vi "main_super.vi"() -> ()   [LabVIEW 2019]
uses:
  Skid_Pump_Water/Padrao_cluster_usuario_entrada_bomba_agua.ctl
  \\SERVERPC\Server/padrao_todos_os_dados_SAIDA.ctl
  \\SERVERPC\Server/padrao_UCM.004.EEL.0300_SAIDA.ctl
  \\SERVERPC\Server/padrao_UCM.004.EEL.0200_SAIDA.ctl
  \\SERVERPC\Server/padrao_INTERNO.ctl
  \\SERVERPC\Server/padrao_ADAM_SAIDA.ctl
  Skid_Pump_Kerosene/Cluster_usuario_entrada_K.ctl
  Skid_Medicao/Padrao_cluster_usuario_entrada(med).ctl
  SkidInjection/Cluster_de_usuario_entrada.ctl
  \\SERVERPC\Server/padrao_tipo_dado.ctl
panel:
  out "KPS-FCV-001-R":dbl
  out "WPS-FCV-001-R":dbl
  out "igual?KMS-EVC-001":bool
  out "igual?WMS-EVC-001B":bool
  out "igual?WMS-EVC-001A":bool
  out "T49 M":bool
  in  "KMS-EVC-001":bool
  out "SKM-FC-KF-AUX 2":bool
  out "T26 K":bool
  in  "KPS-FCV-001-W":i16(slide) scale=0.0..100.0
  out "T24 K":bool
  out "T25 K":bool
  out "igual?AMS-ECV-001A":bool
  out "T26":bool
  in  "WPS-FCV-001-W":i16(slide) scale=0.0..100.0
  out "WPS-FCV-001-AUX":bool
  out "T24":bool
  out "T25":bool
  out "SKM-LAM-CTL":bool
  out "T31 M":bool
  out "T32 M":bool
  out "T30 M":bool
  out "Temperatura":dbl[](array[numeric])
  out "Pressão Diferencial":dbl[](array[numeric])
  out "Pressao Absoluta":dbl[](array[numeric])
  out "SKM-FIC-COR-CTL":bool
  out "igual?AMS-EVC-001C":bool
  out "igual?AMS-EVC-001B":bool
  out "Path":string
  out "Confirma SKM-CV-LAM":bool
  out "Confirma SKM-CV-COR":bool
  out "Confirma caminho 1":bool
  in  "AMS-EVC-001C":bool
  in  "AMS-EVC-001B":bool
  in  "AMS-EVC-001A":bool
  out "SKM-TI-LAM":dbl[](array[numeric])
  in  "Controle ar novo 2":i16(slide) scale=0.0..100.0
  in  "Controle ar novo 1":i16(slide) scale=0.0..100.0
  out "Vazao massica":string
  out "P.dif.":string
  out "P.abs.":string
  out "Temp.":string
  out "SKM-PA-TQ":string
  out "SKM-TI-TQ":string
  out "SKM-PA-BAR":string
  out "SKM-FIM-WF":string
  out "SKM-TI-WF":string
  out "SKI-PD-ST":string
  out "SKM-TI-KF":string
  out "SKM-DEN-COR-KF":string
  out "SKM-TI-COR-KF":string
  out "SKM-FIC-COR-KF":string
  in  "FSS-EVC-803":bool
  in  "FSS-EVC-801":bool
  in  "WPS-EVC-008":bool
  in  "WPS-EVC-007":bool
  in  "WPS-EVC-006":bool
  in  "WPS-EVC-005":bool
  out "tempo-super":dbl
  out "aux4":bool
  out "aux3":bool
  out "aux2":bool
  out "aux1":bool
  out "igual?FSS-EVC-611":bool
  out "igual?FSS-EVC-621":bool
  out "igual?SKS-CV-LT1":bool
  out "igual?SKS-CV-BY1":bool
  out "igual?SKS-CV-LT2":bool
  out "igual?SKS-CV-BY2":bool
  in  "CP-Y-601D":bool caption="SKS-CV-004"
  in  "CP-Y-601H":bool
  out "TM6":bool
  out "FSS-EVC-611":bool
  out "FSS-EVC-621":bool
  out "Maximo  W":bool
  out "Minimo  W":bool
  out "FSS-LSL-621":bool
  out "FSS-LSH-621":bool
  out "FSS-LSA-621":bool
  out "FSS-LIT-801":dbl(slide) scale=0.0..100.0
  out "TM10":bool
  out "TM9":bool
  out "TM8":bool
  in  "FSS-EVC-804":bool
  out "TK6":bool
  out "TW6":bool
  out "TK5":bool
  out "TW5":bool
  out "TM5":bool
  out "TM11":bool
  out "TM7":bool
  out "TM4":bool
  out "TM3":bool
  out "TM2":bool
  out "TM1":bool
  in  "FSS-EVC-802":bool
  out "TK2":bool
  out "TW2":bool
  out "TW4":bool
  out "TK1":bool
  out "TK3":bool
  out "TK4":bool
  out "TW3":bool
  out "TW1":bool
  out "FSS-LSH-611":bool
  out "FSS-LSL-611":bool
  out "Minimo K":bool
  out "Maximo K":bool
  out "FSS-LIT-802":dbl(slide) scale=0.0..100.0
  out "FSS-LSA-611":bool
  out "FSS-LSA-801":bool
  out "igual?SKI-CV-ST":bool
  out "igual?SKI-CV-AR":bool
  out "igual?SKI-CV-KF-ST":bool
  out "igual?SKI-CV-WF-ST":bool
  out "igual?SKI-CV-KF-BY1":bool
  out "igual?SKI-CV-BY2":bool
  out "igual?SKI-CV-WF-BY1":bool
  out "SPK-RD-VEL[%]":dbl
  in  "certificado_SPK-PD-P":bool
  in  "TD-SPK-RD-VEL":bool
  out "SPW-RD-VEL[%]":dbl
  out "T15 K":bool
  out "T14 K":bool
  out "T16 K":bool
  out "T23 K":bool
  out "T11 K":bool
  out "T10 K":bool
  out "T9 K":bool
  out "T13 K":bool
  out "T17 K":bool
  out "T18 K":bool
  out "T12 K":bool
  out "T6 K":bool
  out "T1 K":bool
  out "T19 K":bool
  out "T8 K":bool
  out "T22 K":bool
  out "T21 K":bool
  out "T20 K":bool
  out "T5 K":bool
  out "T4 K":bool
  out "T3 K":bool
  out "T7 K":bool
  out "T2 K":bool
  out "SKI-PD-ST":dbl[](array[numeric])
  out "T20 I":bool
  out "T19 I":bool
  out "T18 I":bool
  out "T17 I":bool
  out "T16 I":bool
  out "T15 I":bool
  out "T14 I":bool
  out "T13 I":bool
  out "T11 I":bool
  out "T12 I":bool
  out "T10 I":bool
  out "T9 I":bool
  out "T8 I":bool
  out "T7 I":bool
  out "T6 I":bool
  out "T4 I":bool
  out "T5 I":bool
  out "T3 I":bool
  out "T2 I":bool
  out "T1 I":bool
  in  "FIS-EVC-001":bool
  in  "FIS-EVC-002":bool
  in  "FIS-EVC-031":bool
  in  "FIS-EVC-021":bool
  in  "FIS-EVC-011":bool
  in  "FIS-EVC-022":bool
  in  "FIS-EVC-012":bool
  out "igual?SKM-FC-AR":bool
  out "igual?AMS-EVC-001E":bool
  in  "TD-SKM-TI-COR-AR":bool
  in  "TD-SKM-DEN-COR-KF":bool
  in  "TD-SKM-PD-LAM":bool
  in  "TD-SKM-TI-COR-KF":bool
  in  "TD-SKM-PA-LAM":bool
  in  "TD-SKM-FIC-COR-KF":bool
  in  "TD-SKM-TI-LAM":bool
  in  "TD-SKM-DEN-COR-AR":bool
  in  "TD-SKM-FIC-COR-AR":bool
  in  "WMS-FCV-001":i16(slide) scale=0.0..100.0
  in  "KMS-FCV-001":i16(slide) scale=0.0..100.0
  in  "AMS-FY-004A":i16(slide) scale=0.0..100.0
  in  "AMS-PY-005A":i16(slide) scale=0.0..100.0
  in  "AMS-EVC-003A":bool
  in  "WMS-EVC-001B":bool
  in  "WMS-EVC-001A":bool
  in  "valvula nova 6":bool
  in  "Controle de vazao novo 2-aux":bool
  in  "valvula nova 5":bool
  in  "valvula nova 4":bool
  in  "valvula nova 3":bool
  in  "WMS-FIT-001B":bool
  in  "controle de vazao novo 1-aux":bool
  in  "TANQUE_AR":bool
  out "SKM-PA-BAR":dbl[](array[numeric])
  out "Vazao Massica Ar":dbl[](array[numeric])
  out "WMS-FIT-001A":dbl[](array[numeric])
  out "WMS-TIT-001":dbl[](array[numeric])
  out "KMS-TIT-003":dbl[](array[numeric])
  out "KMS-TIT-002":dbl[](array[numeric])
  out "SKM-DEN-COR-AR":dbl[](array[numeric])
  out "SKM-TI-COR-AR":dbl[](array[numeric])
  out "SKM-FIC-COR-AR":dbl[](array[numeric])
  out "SKM-PD-LAM":dbl[](array[numeric])
  out "SKM-PA-LAM":dbl[](array[numeric])
  out "AMS-PIT-003":dbl[](array[numeric])
  out "SKM-DEN-COR-KF":dbl[](array[numeric])
  out "SKM-TI-COR-KF":dbl[](array[numeric])
  out "SKM-FIC-COR-KF":dbl[](array[numeric])
  out "SKM-TI-KF-CTL":bool
  out "SKM-TI-WF-CTL":bool
  out "SKM-FC-AR-AUX":bool
  out "SKM-FC-WF-AUX":bool
  out "SKM-FIM-WF-CTL":bool
  out "SKM-FC-KF-AUX":bool
  out "SKM-FIC-COR-KF-CTL":bool
  out "SKM-PC-TQ-AUX":bool
  out "T17 M":bool
  out "T48 M":bool
  out "T20 M":bool
  out "T18 M":bool
  out "T19 M":bool
  out "T21 M":bool
  out "T11 M":bool
  out "T10 M":bool
  out "T28 M":bool
  out "T23 M":bool
  out "T27 M":bool
  out "T26 M":bool
  out "T25 M":bool
  out "T47 M":bool
  out "T46 M":bool
  out "T45 M":bool
  out "T41 M":bool
  out "T42 M":bool
  out "T43 M":bool
  out "T44 M":bool
  out "T40 M":bool
  out "T38 M":bool
  out "T37 M":bool
  out "T39 M":bool
  out "T36 M":bool
  out "T35 M":bool
  out "T33 M":bool
  out "T34 M":bool
  out "T29 M":bool
  out "T24 M":bool
  out "T22 M":bool
  out "T12 M":bool
  out "T16 M":bool
  out "T15 M":bool
  out "T14 M":bool
  out "T13 M":bool
  out "T9 M":bool
  out "T8 M":bool
  out "T6 M":bool
  out "T7 M":bool
  out "T5 M":bool
  out "T4 M":bool
  out "T2 M":bool
  out "T3 M":bool
  out "T1 M":bool
  out "igual?SPK-WR-VEL":bool
  out "igual?SPK-WR-ON":bool
  out "igual?SPK-WR-OFF":bool
  out "igual?PID-KF-ON":bool
  out "igual?SPK-CV-008":bool
  out "igual?SPK-CV-007":bool
  out "igual?SPK-CV-006":bool
  out "igual?SPK-CV-005":bool
  out "igual?SPK-CV-004":bool
  out "igual?SPK-CV-003":bool
  out "igual?SPK-CV-002":bool
  out "igual?SPK-CV-001":bool
  in  "SPK-WR-VEL":i32(slide) scale=0.0..100.0
  out "SPK-RD-VEL":dbl(knob) scale=0.0..3500.0
  out "SPK-PD-P":dbl
  out "SPK-RD-TU":dbl
  out "SPK-RD-CRT":dbl
  out "SPK-RD-IA":dbl
  out "SPK-RD-ST":dbl
  out "Inversor Desligado":bool
  out "Inversor Ligado":bool
  out "Bomba K":bool
  in  "PID-KF-ON":bool=TRUE
  in  "KPS-WR-OFF":bool
  in  "KPS-WR-ON":bool
  in  "KPS-EVC-006":bool
  in  "KPS-EVC-005":bool
  in  "KPS-EVC-007":bool
  in  "KPS-EVC-008":bool
  in  "KPS-EVC-003":bool
  in  "KPS-EVC-004":bool
  in  "KPS-EVC-002":bool
  in  "KPS-EVC-001":bool
  out "T15":bool
  out "T14":bool
  out "T16":bool
  out "T23":bool
  out "T11":bool
  out "T10":bool
  out "T9":bool
  out "T13":bool
  out "T17":bool
  out "T18":bool
  out "T12":bool
  out "T6":bool
  out "T1":bool
  out "T19":bool
  out "T8":bool
  out "T22":bool
  out "T21":bool
  out "T20":bool
  out "T5":bool
  out "T4":bool
  out "T3":bool
  out "T7":bool
  out "T2":bool
  out "Inversor desligado":bool
  out "Inversor ligado":bool
  out "Bomba W":bool
  out "igual?SPW-WR-VEL":bool
  out "igual?PID-WF-ON":bool
  out "igual?WPS-EVC-003":bool
  out "igual?WPS-EVC-007":bool
  out "igual?WPS-EVC-006":bool
  out "igual?SPW-WR-OFF":bool
  out "igual?SPW-WR-ON":bool
  out "igual?WPS-EVC-008":bool
  out "igual?WPS-EVC-005":bool
  out "igual?WPS-EVC-004":bool
  out "igual?WPS-EVC-002":bool
  out "igual?WPS-EVC-001":bool
  in  "certificado_SPW-PD-P":bool
  in  "TD-SPW-RD-VEL":bool
  out "SPW-PD-P":dbl
  out "SPW-RD-TU":dbl
  out "SPW-RD-CRT":dbl
  out "SPW-RD-IA":dbl
  out "SPW-RD-ST":dbl
  out "SPW-RD-VEL":dbl(knob) scale=0.0..3500.0
  in  "WPS-EVC-001":bool
  in  "WPS-EVC-004":bool
  in  "PID-WF-ON":bool=TRUE
  in  "WPS-WR-OFF":bool
  in  "WPS-WR-ON":bool
  in  "SPW-WR-VEL":i32(slide) scale=0.0..100.0
  in  "WPS-EVC-003":bool
  in  "WPS-EVC-002":bool
  in  "[ESC/STOP]":bool
  out "Comunicacao Server Client":bool
  out "Status_Comunicacao":string
  in  "Abrir Editor Prioridade":bool
  out "RODANDO TESTE ??":bool
  out "Separador":bool
  # "ALL SKIDS"
  # "MAIN"
  # "[rpm]"
  # "[rpm]"
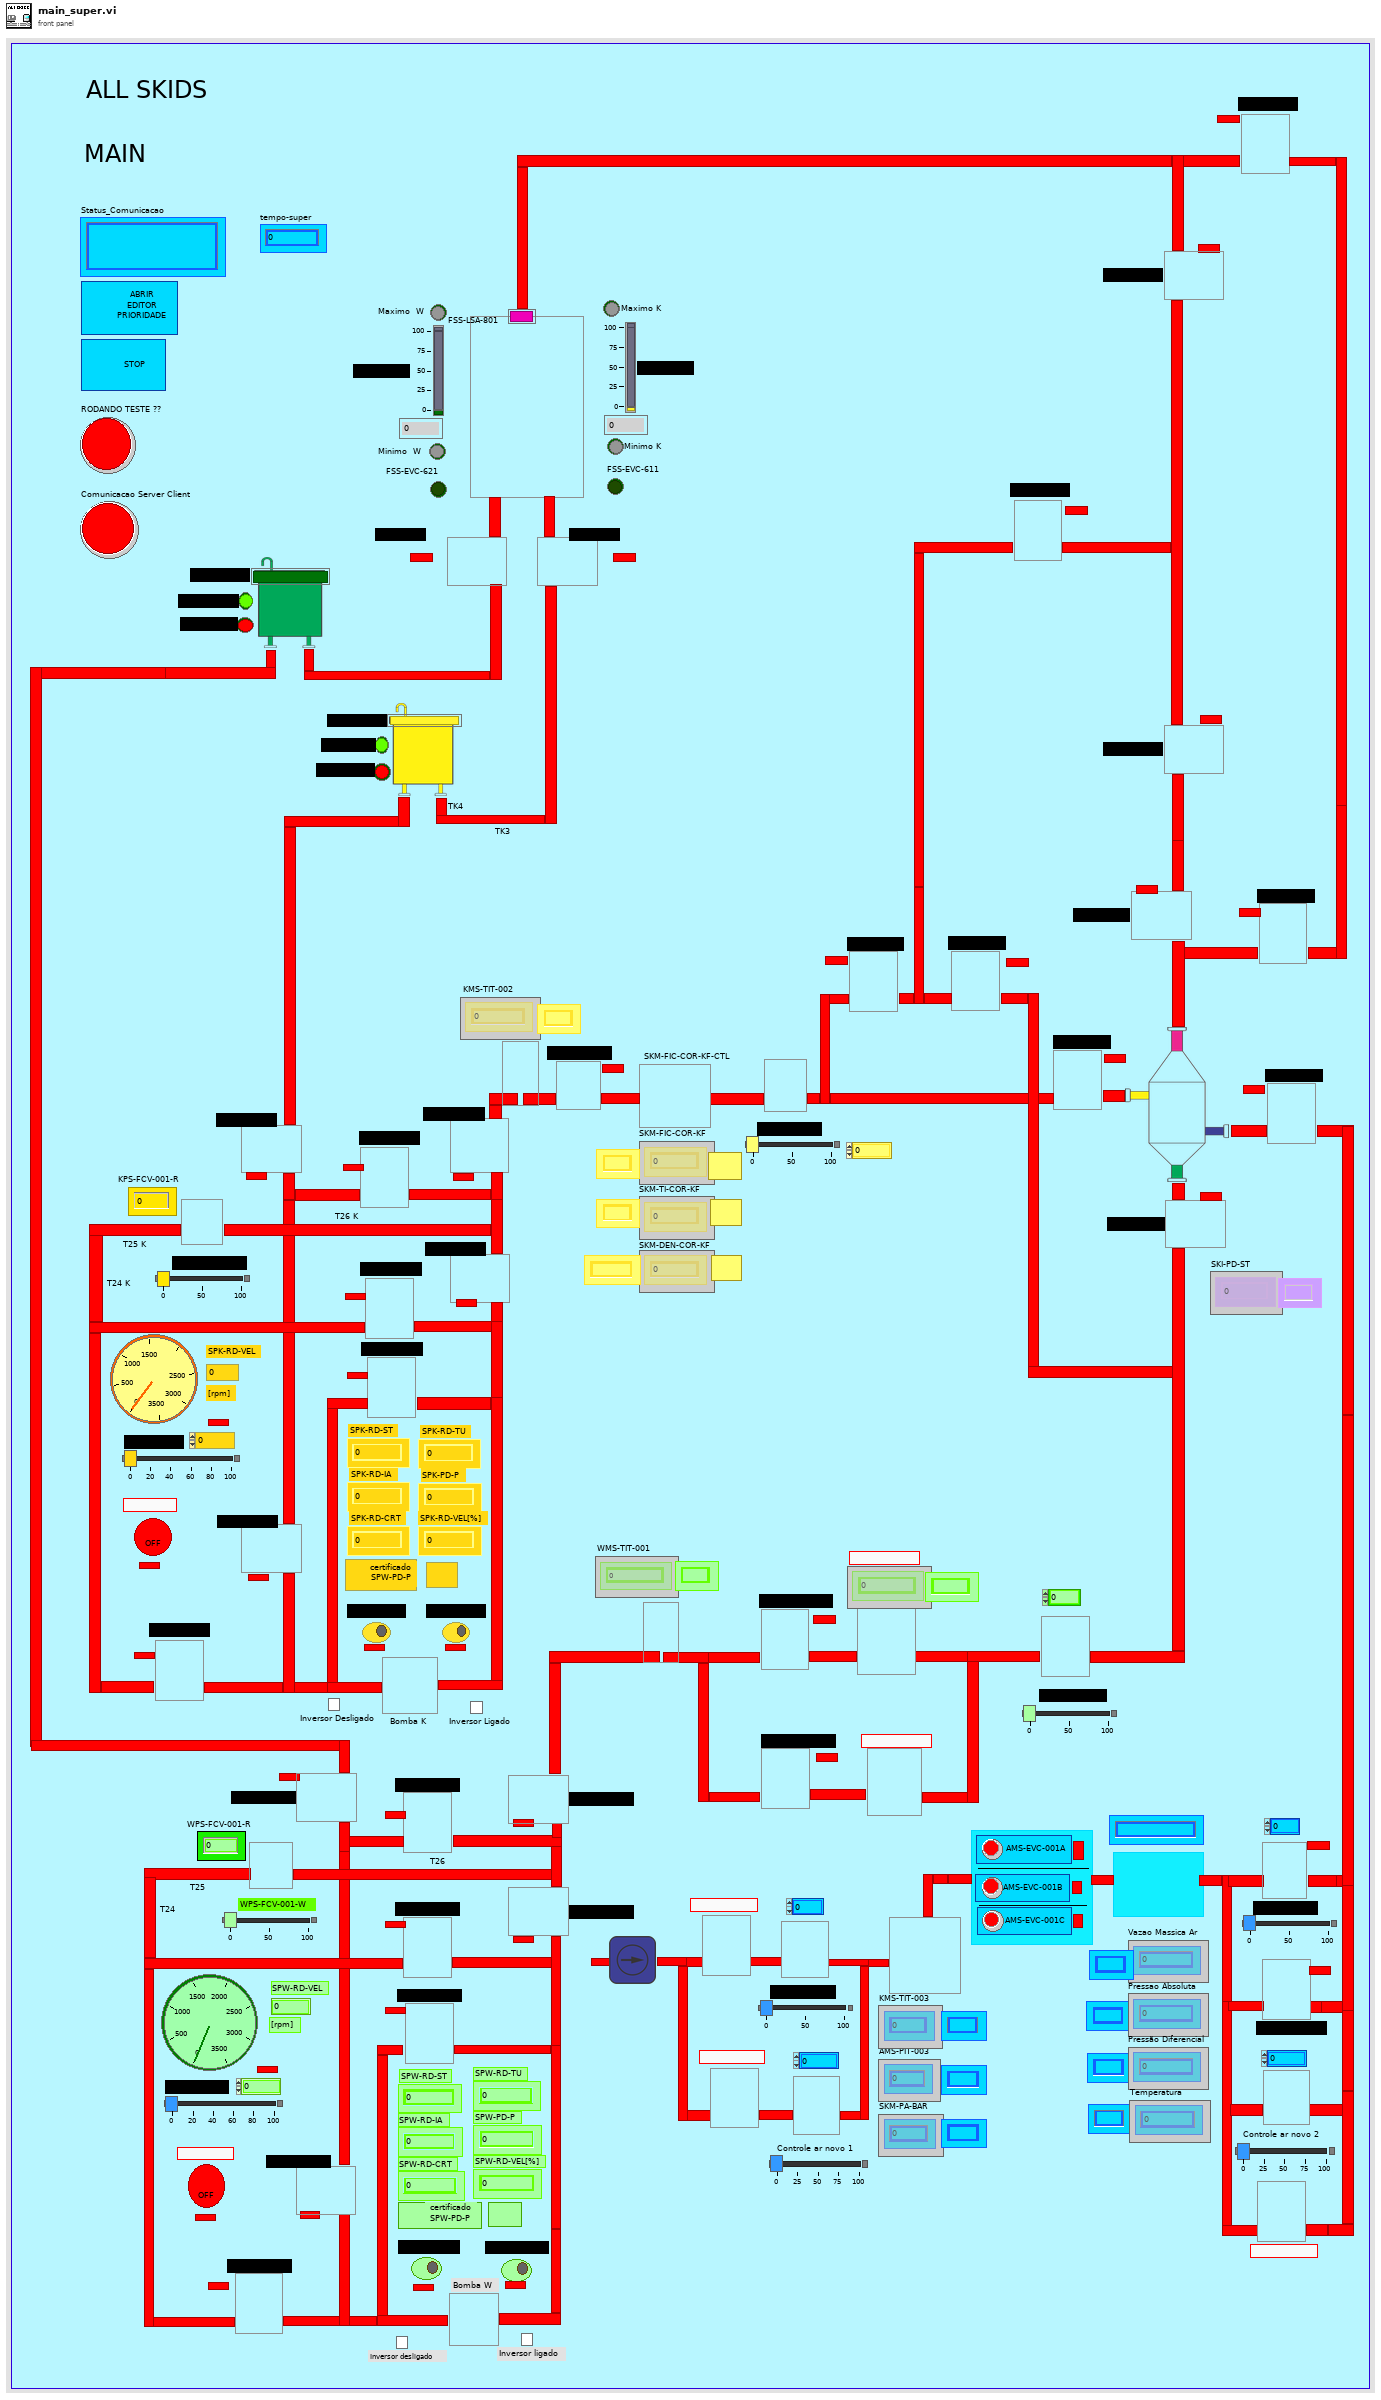
[diagram p1: front panel]
types:
  T1 = typedef "Cluster_de_usuario_entrada.ctl" = cluster{"VI USUARIO":path, "Tipo de Dado_C":T2, "Certificado":bool}
  T2 = typedef "padrao_tipo_dado.ctl" = u16
  T3 = typedef "padrao_todos_os_dados_SAIDA.ctl" = cluster{"UCM.004.EEL.0300_SAIDA":T4, "UCM.004.EEL.0200_SAIDA":T5, "INTERNO":T6, "ADAM_SAIDA":T7}
  T4 = typedef "padrao_UCM.004.EEL.0300_SAIDA.ctl" = cluster{"DIGITAL":cluster{"KPS-EVC-001":bool, "KPS-EVC-002":bool, "KPS-EVC-003":bool, "KPS-EVC-004":bool, "KPS-EVC-005":bool, "KPS-EVC-006":bool, "KPS-EVC-007":bool, "KPS-EVC-008":bool, "WPS-EVC-001":bool, "WPS-EVC-002":bool, "WPS-EVC-003":bool, "WPS-EVC-004":bool, "WPS-EVC-005":bool, "WPS-EVC-006":bool, "WPS-EVC-007":bool, "WPS-EVC-008":bool, "AMS-EVC-001B":bool, "AMS-EVC-003A":bool, "FIS-EVC-031":bool, "FIS-EVC-011":bool, "FIS-EVC-012":bool, "FIS-EVC-021":bool, "FIS-EVC-022":bool, "FIS-EVC-001":bool, "FIS-EVC-002":bool, "KMS-EVC-001":bool, "WMS-EVC-001A":bool, "WMS-EVC-001B":bool, "AMS-EVC-001C":bool, "DG-EVC-001":bool, "DG-EVC-ALL":bool, "PID-PC-TQ-ON":bool, "PID-FC-AR-ON":bool, "PID-WF-ON":bool, "PID-KF-ON":bool, "PID-SA-WF-INV":bool, "PID-SA-KF-INV":bool, "PID-SA-AR-COR":bool, "KPS-WR-ON":bool, "WPS-WR-ON":bool, "KPS-WR-OFF":bool, "WPS-WR-OFF":bool, "AMS-EVC-001A":bool}, "ANALOGICO":cluster{"AMS-PY-005A":i16, "AMS-FY-004A":i16, "WMS-FCV-001":i16, "KMS-FCV-001":i16, "X33 5":i16, "X33 6":i16, "X33 7":i16, "X33 8":i16, "X33 9":i16, "X33 10":i16, "X33 11":i16, "X33 12":i16, "X33 13":i16, "X33 14":i16, "PID-PC-TQ-SP":i16, "PID-FC-AR-SP":i16, "PID-FC-WF-SP":i16, "PID-FC-KF-SP":i16, "PID-INC-WF-SP":i16, "PID-INC-KF-SP":i16, "SPK-WR-VEL":i32, "SPW-WR-VEL":i32, "SKM-FIC-COR-KF-MAX":dbl, "SKM-FIC-COR-KF-MIN":dbl, "SKM-FIC-COR-WF-MAX":dbl, "SKM-FIC-COR-WF-MIN":dbl, "PID-PC-TQ-GP":dbl, "PID-PC-TQ-GI":dbl, "PID-PC-TQ-GD":dbl, "PID-FC-AR-GP":dbl, "PID-FC-AR-GI":dbl, "PID-FC-AR-GD":dbl, "PID-FC-WF-GP":dbl, "PID-FC-WF-GI":dbl, "PID-FC-WF-GD":dbl, "PID-FC-KF-GP":dbl, "PID-FC-KF-GI":dbl, "PID-FC-KF-GD":dbl, "PID-INV-WF-GP":dbl, "PID-INV-WF-GI":dbl, "PID-INV-WF-GD":dbl, "PID-INV-KF-GP":dbl, "PID-INV-KF-GI":dbl, "PID-INV-KF-GD":dbl}}
  T5 = typedef "padrao_UCM.004.EEL.0200_SAIDA.ctl" = cluster{"DIGITAL":cluster{"FSS-EVC-801":bool, "FSS-EVC-802":bool, "FSS-EVC-803":bool, "CP-Y-601D":bool, "CP-Y-601H":bool, "FSS-EVC-804":bool, "SHD-CV-HD":bool, "SHD-CV-ALV":bool, "SHD-ON-OFF":bool, "FSS-EVC-805":bool, "FSS-EVC-806":bool, "X31-12":bool, "X31-13":bool, "X31-14":bool, "X31-15":bool, "X31-16":bool}, "ANALOGICO":cluster{"DG-FCV-801":i16, "X33-2":i16, "FRAM-1100":i16}}
  T6 = typedef "padrao_INTERNO.ctl" = cluster{"DIGITAL":cluster{"ITN-SI-SS-1":bool, "ITN-SI-SS-2":bool, "ITN-SI-SS-3":bool, "ITN-SS-SW-1":bool, "ITN-SS-SK-1":bool, "ITN-SPW-SKM":bool, "ITN-SKMW-SI":bool, "ITN-SKMK-SI":bool, "ITN-SKMA-SI":bool, "ITN-SPK-SKM":bool, "Aplicação apenas de Leitura ??":bool, "SALVAR/AQUISITAR":bool}, "ANALOGICO":cluster{"ITN_Vazao_Massica_Ar":dbl[], "ITN_Vazao_Volumetrica_WF":dbl[], "ITN_Vazao_Massica_KF":dbl[], "ITN_Vazao_Massica_WF":dbl[], "ITN_Vazao_Volumetrica_KF":dbl[], "ITN_Temperatura":dbl[], "ITN_Pressão_Absoluta":dbl[], "ITN_Pressão_Diferencial":dbl[]}, "ALARMES-INTERNOS":cluster{"ALR-AMS-001A+B":bool, "ALR-AMS-001A+C":bool, "ALR-AMS-001B+C":bool, "ALR-AMS-001A+B+C":bool, "ALR-WMS-001A+B":bool}}
  T7 = typedef "padrao_ADAM_SAIDA.ctl" = cluster{"DIGITAL":cluster{"KPS-FCV-001-W":dbl, "WPS-FCV-001-W":dbl, "ADAM-4024-W-2":dbl, "ADAM-4024-W-3":dbl}}
  T8 = typedef "Padrao_cluster_usuario_entrada(med).ctl" = cluster{"VI USUARIO":path, "certificado_SKM-PC-TQ":bool, "certificado_SKM-CV-COR":bool, "certificado_SKM-CV-LAM":bool, "certificado_SKM-CV-JMP":bool, "certificado_SKM-FC-KF":bool, "certificado_SKM-FIC-COR-KF ":bool, "certificado_SKM-FC-WF":bool, "certificado_SKM-FIM-WF":bool, "certificado_SKM-TI-KF":bool, "certificado_SKM-TI-WF":bool, "TD-SKM-TI-COR-AR":bool, "TD-SKM-FIC-COR-AR":bool, "TD-SKM-DEN-COR-AR":bool, "TD-SKM-TI-LAM":bool, "TD-SKM-FIC-COR-KF":bool, "TD-SKM-PA-LAM":bool, "TD-SKM-TI-COR-KF":bool, "TD-SKM-PD-LAM":bool, "TD-SKM-DEN-COR-KF":bool, "certificado_SKM-PA-LAM":bool, "certificado_SKM-PD-LAM":bool, "certificado_SKM-TI-LAM":bool, "certificado_SKM-FIC-COR-AR":bool, "certificado_SKM-PA-BAR":bool}
  T9 = typedef "Cluster_usuario_entrada_K.ctl" = cluster{"File Path Control":path, "certificado_SPK-PD-P":bool, "TD-SPK-RD-VEL":bool, "TD-SPK-RD-IA":bool, "TD-SPK-RD-CRT":bool, "TD-SPK-RD-TU":bool, "TD-SPK-PD-P":bool, "TD-SPK-RD-ST":bool}
  T10 = typedef "Padrao_cluster_usuario_entrada_bomba_agua.ctl" = cluster{"Path Main":path, "certificado_SPW-PD-P":bool, "TD-SPW-RD-VEL":bool, "TD-SPW-RD-IA":bool, "TD-SPW-RD-CRT":bool, "TD-SPW-RD-TU":bool, "TD-SPW-PD-P":bool, "TD-SPW-RD-ST":bool}
  T11 = typedef "padrao_todos_os_dados_ENTRADA.ctl" = cluster{"PAINEL_ADAM_ENTRADA":T12, "todos_os_dados_SAIDA":T3, "UCM.004.EEL.0300_ENTRADA":T13, "UCM.004.EEL.0200_ENTRADA":T14}
  T12 = typedef "padrao_ADAM_ENTRADA.ctl" = cluster{"ANALOGICO":cluster{"KPS-FCV-001-R":dbl, "WPS-FCV-001-R":dbl, "ADAM-4017-01-02":dbl, "ADAM-4017-01-03":dbl, "ADAM-4017-01-04":dbl, "ADAM-4017-01-05":dbl, "ADAM-4017-01-06":dbl, "ADAM-4017-01-07":dbl}, "Laminador_Omega":cluster{"Mode ":string, "Abs. Pressure ":dbl, "Mass Flow":dbl, "Temperature":dbl, "Volumetric Flow":dbl, "Substance ":string}}
  T13 = typedef "padrao_UCM.004.EEL.0300_ENTRADA.ctl" = cluster{"DIGITAL":cluster{"ADAM-ON":bool, "CLP-ON":bool, "KMS-ZT-001":bool, "WMS-ZT-001A":bool, "WMS-ZT-001B":bool, "AMS-ZT-001A":bool, "AMS-ZT-001B":bool, "AMS-ZT-001C":bool, "AMS-ZT-003A":bool, "DG-ZT-001":bool, "DG-ZT-201A":bool, "DG-ZT-201B":bool, "DG-ZT-ON":bool, "DG-ZT-201":bool, "DG-ZT-501":bool, "DG-ZT-701":bool, "KPS-RD-ALR":bool, "KPS-RD-VVT":bool, "KPS-RD-FLL":bool, "WPS-RD-ALR":bool, "WPS-RD-VVT":bool, "WPS-RD-FLL":bool}, "ANALOGICO":cluster{"AMS-PIT-001":dbl[], "AMS-PIT-005":dbl[], "AMS-TIT-005":dbl[], "AMS-PIT-004A":dbl[], "AMS-TIT-004":dbl[], "AMS-PDIT-004A":dbl[], "WMS-TIT-001":dbl[], "WMS-FIT-001B":dbl[], "X32 09":dbl[], "AMS-FIT-004B":dbl[], "WPS-VMS-001":dbl[], "KPS-VMS-001":dbl[], "KMS-TIT-002":dbl[], "WPS-PD-001":dbl[], "KPS-PD-001":dbl[], "X32 16 ":dbl[], "X32 17":dbl[], "X32 18":dbl[], "X32 19":dbl[], "X32 20":dbl[], "X32 21":dbl[], "X32 22":dbl[], "X32 23":dbl[], "X32 24":dbl[], "KPS-RD-ST":dbl[], "WPS-RD-ST":dbl[], "KPS-RD-VEL":dbl[], "WPS-RD-VEL":dbl[], "KPS-RD-IA":dbl[], "WPS-RD-IA":dbl[], "KPS-RD-TU":dbl[], "WPS-RD-TU":dbl[], "KMS-FIT-TI-001":dbl[], "KMS-FIT-DEN-001":dbl[], "KMS-FIT-FIC-001":dbl[], "WMS-FIT-TI-001A":dbl[], "WMS-FIT-DEN-001A":dbl[], "KPS-RD-CRT":dbl[], "WPS-RD-CRT":dbl[], "WMS-FIT-FIC-001A":dbl[]}}
  T14 = typedef "padrao_UCM.004.EEL.0200_ENTRADA.ctl" = cluster{"DIGITAL":cluster{"FSS-LSA-801":bool, "FSS-LSA-621":bool, "FSS-LSA-611":bool, "FSS-LSL-621":bool, "FSS-LSH-621":bool, "FSS-LSL-611":bool, "FSS-LSH-611":bool, "CLP-601-ON":bool, "FSS-ZT-611":bool, "FSS-ZT-621":bool, "X30-11":bool, "X30-12":bool, "DG-ZT-501A":bool, "DG-ZT-501B":bool, "DG-ZT-701A":bool, "DG-ZT-701B":bool}, "ANALOGICO":cluster{"FSS-LIT-802":dbl[], "FSS-LIT-801":dbl[], "SHD-TI-AMB":dbl[], "X32-4":dbl[], "SHD-PD-HD":dbl[], "SHD-PA-JG":dbl[], "X32-7":dbl[], "FRAM-2925":dbl[], "FRAM-2975":dbl[], "FRAM-2976":dbl[], "FRAM-2977":dbl[], "FRAM-2978":dbl[], "FRAM-2979":dbl[], "FRAM-2980":dbl[], "FRAM-2981":dbl[], "FRAM-2982":dbl[], "FRAM-2983":dbl[], "FRAM-2984":dbl[], "FRAM-2985":dbl[], "FRAM-2986":dbl[], "FRAM-2987":dbl[]}}
  T15 = cluster{"igual?SPK-CV-001":bool, "igual?SPK-CV-002":bool, "igual?SPK-CV-003":bool, "igual?SPK-CV-004":bool, "igual?SPK-CV-005":bool, "igual?SPK-CV-006":bool, "igual?SPK-CV-007":bool, "igual?SPK-CV-008":bool, "igual?PID-KF-ON":bool, "igual?SPK-WR-OFF":bool, "igual?SPK-WR-ON":bool, "igual?SPK-WR-VEL":bool, "igual?KPS-FCV-001":bool}
  T16 = typedef "Cluster_usuario_saida_K.ctl" = cluster{"Tubos":cluster{"T1":bool, "T2":bool, "T3":bool, "T4":bool, "T5":bool, "T6":bool, "T7":bool, "T8":bool, "T9":bool, "T10":bool, "T11":bool, "T12":bool, "T13":bool, "T14":bool, "T15":bool, "T16":bool, "T17":bool, "T18":bool, "T19":bool, "T20":bool, "T21":bool, "T22":bool, "T23":bool, "T24":bool, "T25":bool, "T26":bool}, "Leitura_INV":cluster{"SPK-RD-ST":dbl, "SPK-RD-VEL":dbl, "SPK-RD-IA":dbl, "SPK-RD-CRT":dbl, "SPK-RD-TU":dbl, "SPK-PD-P":dbl}, "Inversor":cluster{"Bomba":bool, "Inversor Ligado":bool, "Inversor Desligado":bool}, "Aux":cluster{"SKM-FC-KF-AUX":bool}}
  T17 = cluster{"igual?SPW-CV-001":bool, "igual?SPW-CV-002":bool, "igual?SPW-CV-003":bool, "igual?SPW-CV-004":bool, "igual?SPW-CV-005":bool, "igual?SPW-CV-006":bool, "igual?SPW-CV-007":bool, "igual?SPW-CV-008":bool, "igual?SPW-WR-ON":bool, "igual?SPW-WR-OFF":bool, "igual?PID-WF-ON":bool, "igual?SPW-WR-VEL":bool, "igual?WPS-FVC-001":bool}
  T18 = typedef "Padrao_cluster_usuario_saida_bomba_agua.ctl" = cluster{"Tubos":cluster{"T1":bool, "T2":bool, "T3":bool, "T4":bool, "T5":bool, "T6":bool, "T7":bool, "T8":bool, "T9":bool, "T10":bool, "T11":bool, "T12":bool, "T13":bool, "T14":bool, "T15":bool, "T16":bool, "T17":bool, "T18":bool, "T19":bool, "T20":bool, "T21":bool, "T22":bool, "T23":bool, "T24":bool, "T25":bool, "T26":bool}, "Leitura_INV":cluster{"SPW-RD-ST":dbl, "SPW-RD-VEL":dbl, "SPW-RD-IA":dbl, "SPW-RD-CRT":dbl, "SPW-RD-TU":dbl, "SPW-PD-P":dbl}, "Inversor":cluster{"Bomba":bool, "Inversor Ligado":bool, "Inversor Desligado":bool}, "Aux":cluster{"WPS-FCV-001-AUX":bool}}
  T19 = typedef "Padrao_cluster_usuario_saida_medicao.ctl" = cluster{"Tubos":cluster{"T1":bool, "T2":bool, "T3":bool, "T4":bool, "T5":bool, "T6":bool, "T7":bool, "T8":bool, "T9":bool, "T10":bool, "T11":bool, "T12":bool, "T13":bool, "T14":bool, "T15":bool, "T16":bool, "T17":bool, "T18":bool, "T19":bool, "T20":bool, "T21":bool, "T22":bool, "T23":bool, "T24":bool, "T25":bool, "T26":bool, "T27":bool, "T28":bool, "T29":bool, "T30":bool, "T31":bool, "T32":bool, "T33":bool, "T34":bool, "T35":bool, "T36":bool, "T37":bool, "T38":bool, "T39":bool, "T40":bool, "T41":bool, "T42":bool, "T43":bool, "T44":bool, "T45":bool, "T46":bool, "T47":bool, "T48":bool, "T49":bool}, "Variaveis leitura rapida":cluster{"AMS-PIT-003":dbl[], "SKM-PA-LAM":dbl[], "SKM-TI-LAM":dbl[], "SKM-PD-LAM":dbl[], "WMS-FIT-TI-001A":dbl[], "WMS-FIT-DEN-001A":dbl[], "WMS-FIT-FIC-001A":dbl[], "KMS-FIT-TI-001":dbl[], "KMS-FIT-DEN-001":dbl[], "KMS-FIT-FIC-001":dbl[], "WMS-TIT-001":dbl[], "KMS-TIT-002":dbl[], "KMS-TIT-003":dbl[], "WMS-FIT-001A":dbl[], "Vazao Massica Ar":dbl[], "SKM-PA-BAR":dbl[], "Temperatura":dbl[], "Pressão Absoluta ":dbl[], "Pressão Diferencial":dbl[]}, "Aux":cluster{"SKM-FC-WF-AUX":bool, "SKM-FC-KF-AUX":bool, "SKM-PC-TQ-AUX":bool, "SKM-FC-AR-AUX":bool, "SKM-FIM-WF-CTL":bool, "SKM-FIC-COR-CTL":bool, "SKM-FIC-COR-KF-CTL":bool, "SKM-LAM-CTL":bool, "SKM-TI-KF-CTL":bool, "SKM-TI-TQ-CTL":bool, "SKM-TI-WF-CTL":bool}}
  T20 = cluster{"igual?SKM-FC-WF":bool, "igual?SKM-FC-KF":bool, "igual?SKM-PC-TQ":bool, "igual?SKM-CV-COR":bool, "igual?SKM-CV-LAM":bool, "igual?SKM-CV-JMP":bool, "igual?SKM-FC-AR":bool, "igual?WMS-EVC-001A":bool, "igual?WMS-EVC-001B":bool, "igual?KMS-EVC-001":bool}
  T21 = typedef "Cluster_de_usuario_saida.ctl" = cluster{"Tubos":cluster{"T1":bool, "T 2":bool, "T 3":bool, "T 4":bool, "T 5":bool, "T 6":bool, "T 7":bool, "T 8":bool, "T 9":bool, "T 10":bool, "T 11":bool, "T 12":bool, "T 13":bool, "T 14":bool, "T 15":bool, "T 16":bool, "T 17":bool, "T 18":bool, "T 19":bool, "T 20":bool}, "Leitura":cluster{"SKI-PD-ST":dbl[]}}
  T22 = cluster{"igual?SKI-CV-AR":bool, "igual?SKI-CV-KF-ST":bool, "igual?SKI-CV-KF-BY1":bool, "igual?SKI-CV-WF-ST":bool, "igual?SKI-CV-WF-BY1":bool, "igual?SKI-CV-ST":bool, "igual?SKI-CV-BY2":bool}
  T23 = cluster{"Igual?SKS-CV-BY1":bool, "Igual?SKS-CV-BY2":bool, "Igual?SKS-CV-LT2":bool, "Igual?SKS-CV-TSW":bool, "Igual?SKS-CV-TSK":bool, "Igual?SKS-CV-LT1":bool}
  T24 = cluster{"FSS-LSA-801":bool, "FSS-LSA-621":bool, "FSS-LSA-611":bool, "FSS-LSL-621":bool, "FSS-LSH-621":bool, "FSS-LSL-611":bool, "FSS-LSH-611":bool, "TW2 ":bool, "TK2":bool, "TM5":bool, "TM6":bool, "TM7":bool, "TM8":bool, "TM9":bool, "TM11":bool, "FSS-LIT-801":dbl, "FSS-LIT-802":dbl, "TM10":bool, "Valor minimo atingido K":bool, "Valor maximo atingido K":bool, "Valor maximo atingido W":bool, "Valor minimo atingido W":bool, "TK1":bool, "TW3":bool, "TW4":bool, "TW5":bool, "TW6 ":bool, "TK3":bool, "TK4":bool, "TK5":bool, "TK6":bool, "TM4":bool, "TW1":bool, "FSS-EVC-621":bool, "FSS-EVC-611":bool, "SKS-CV-LT2":bool, "SKS-CV-LT1":bool, "SKS-CV-BY1":bool, "SKS-CV-BY2":bool, "TM1":bool, "TM2":bool, "TM3":bool}
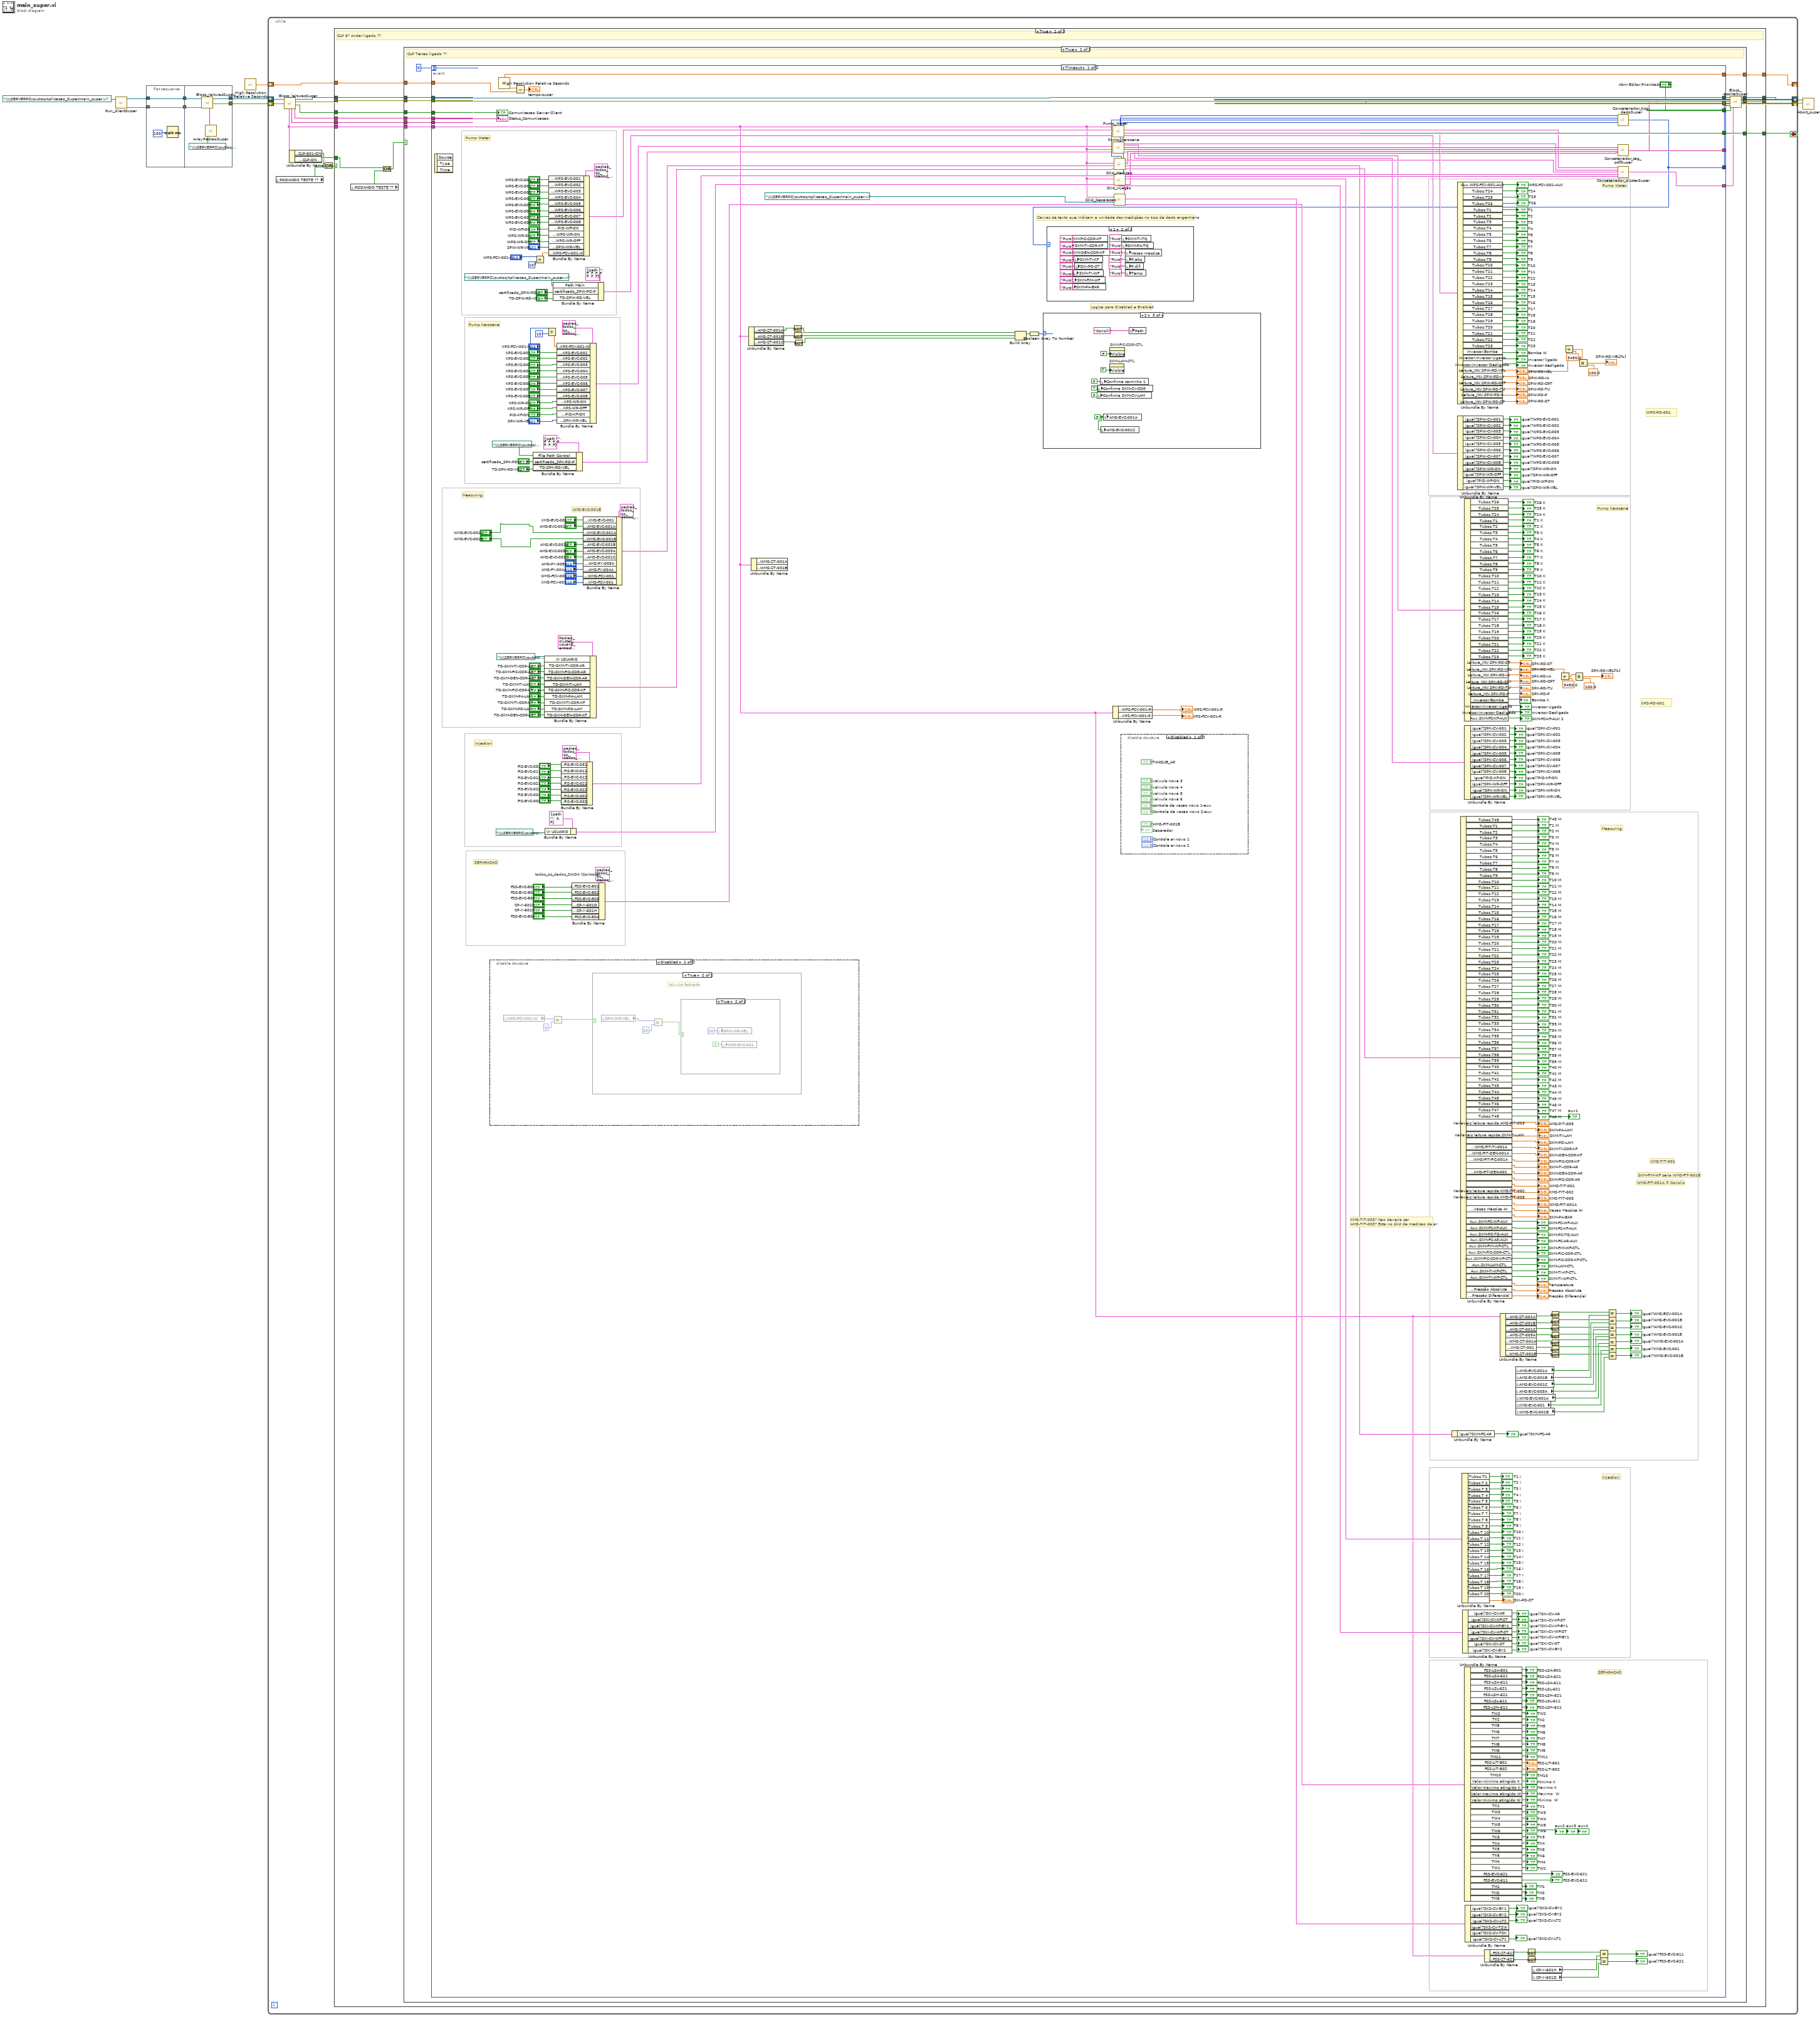
[diagram p0: block diagram]
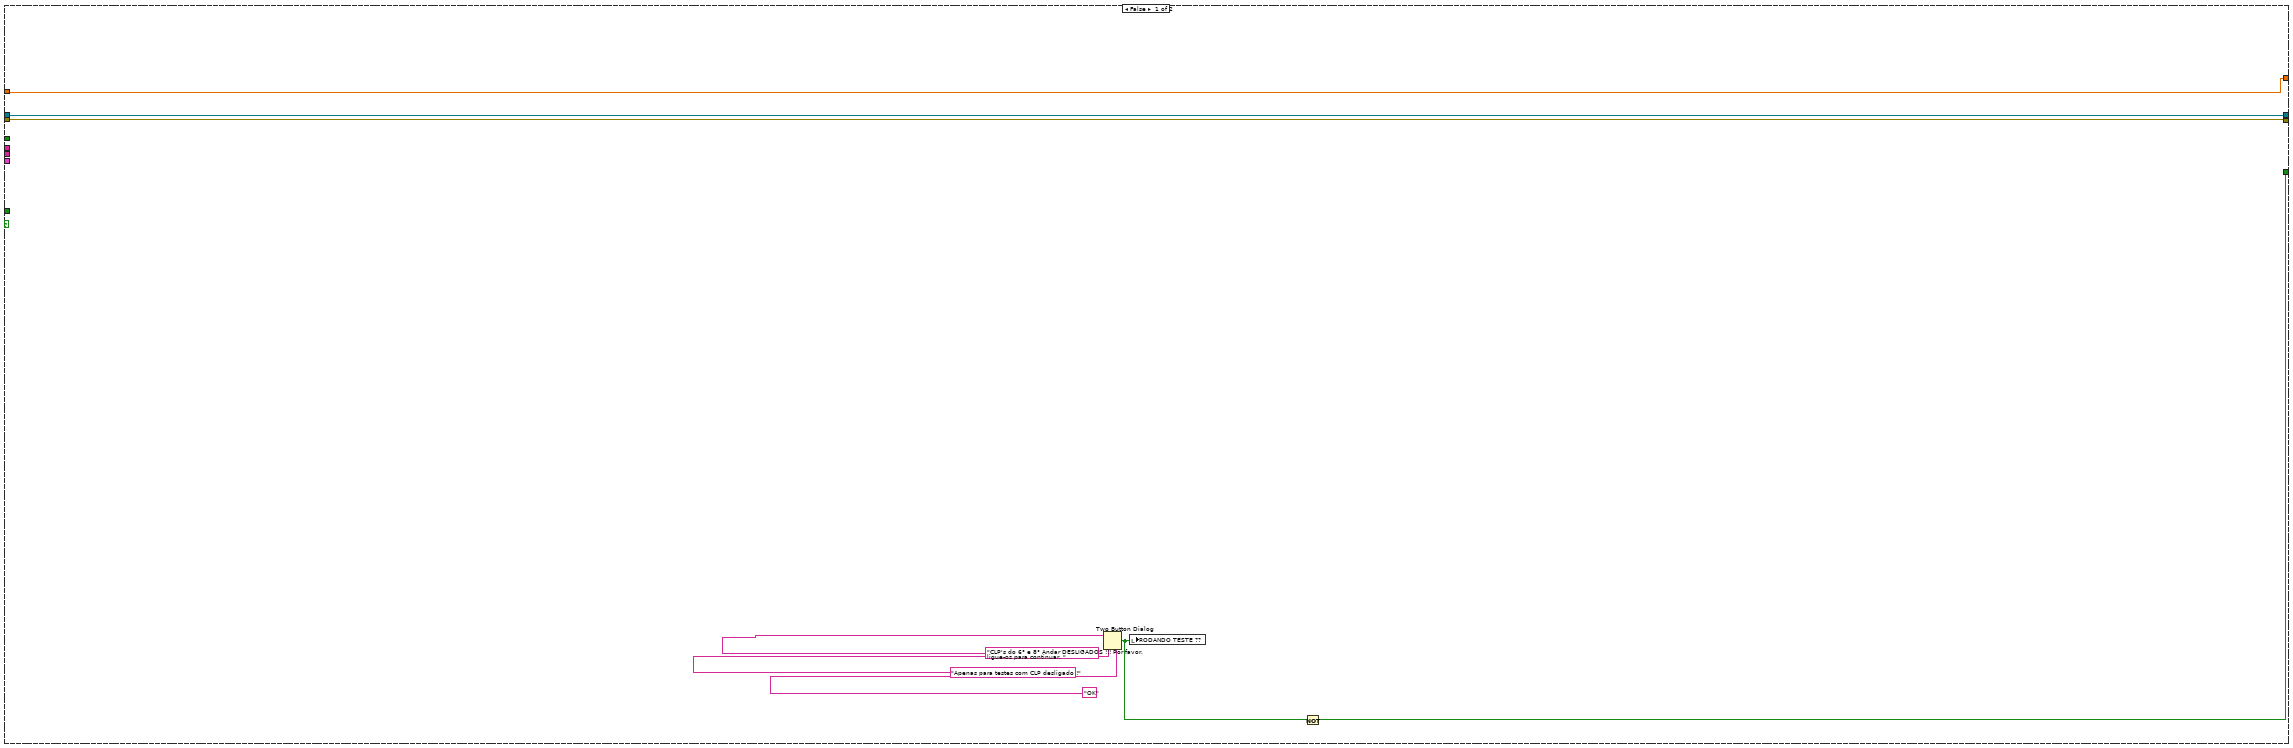
[diagram p2: hidden frame]
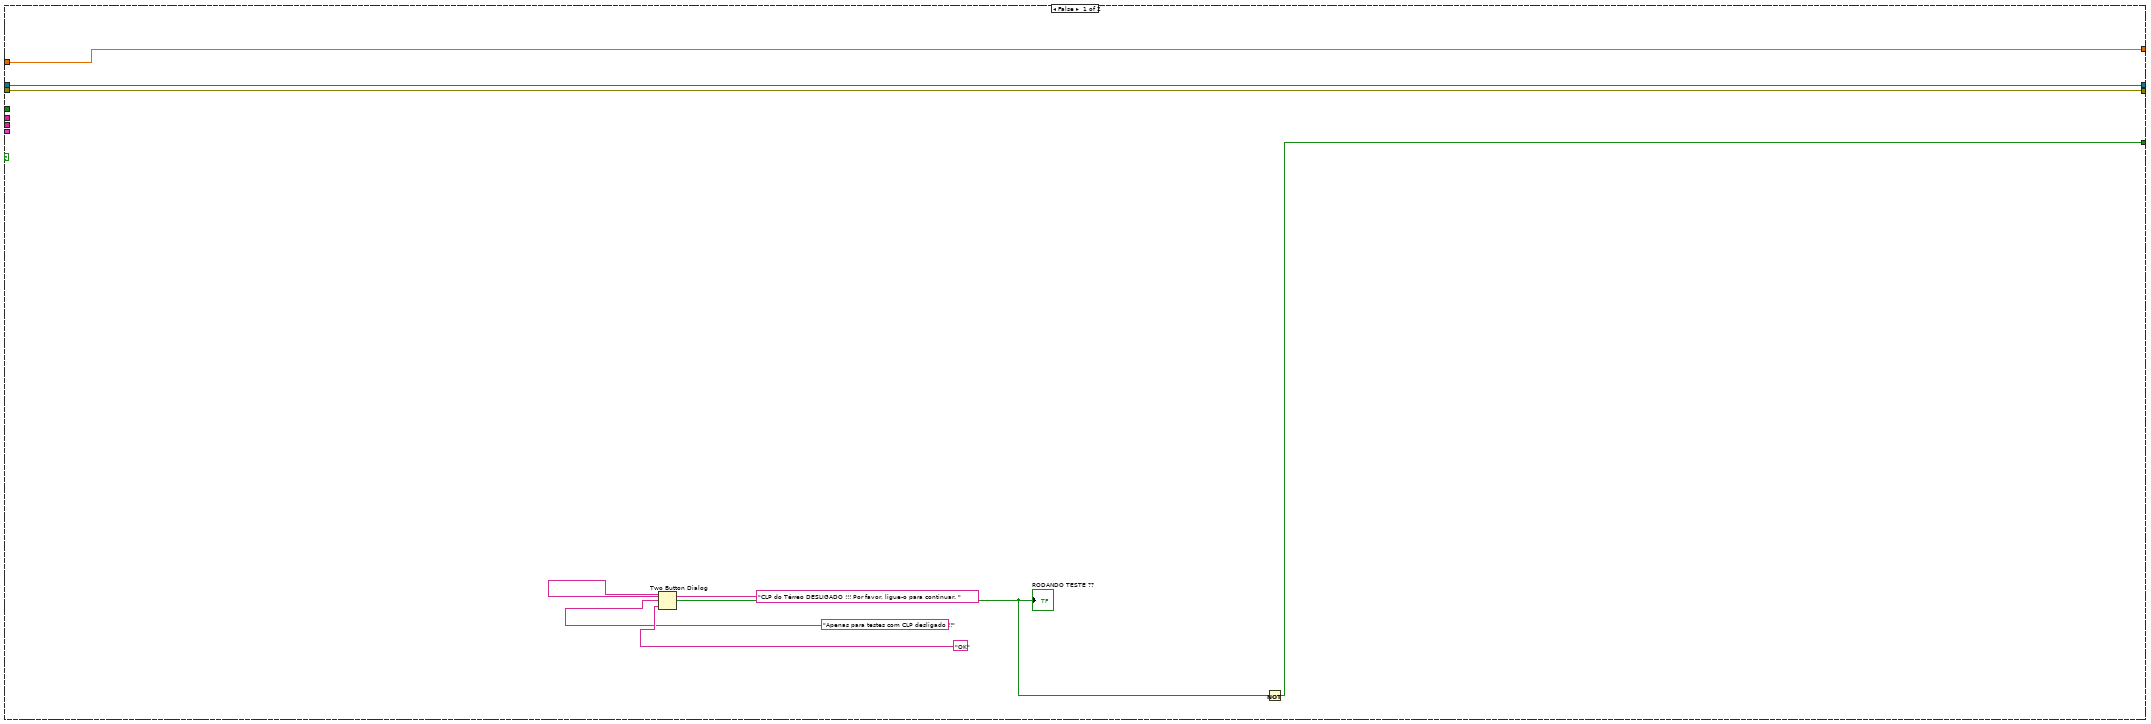
[diagram p3: hidden frame]
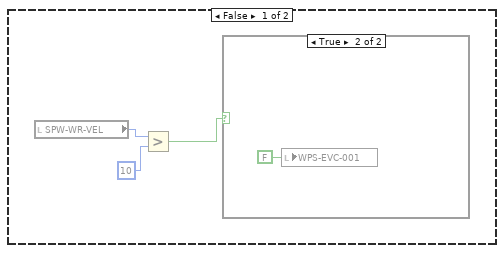
[diagram p4: hidden frame]
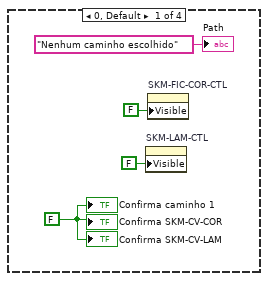
[diagram p8: hidden frame]
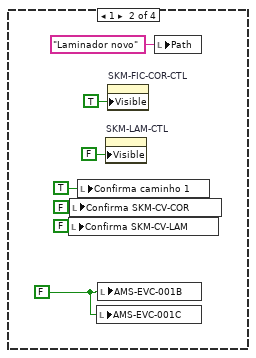
[diagram p9: hidden frame]
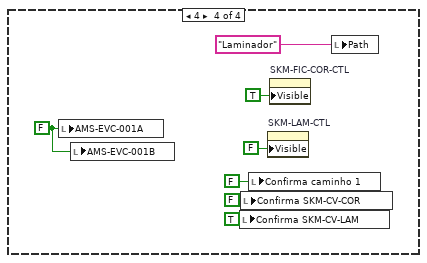
[diagram p10: hidden frame]
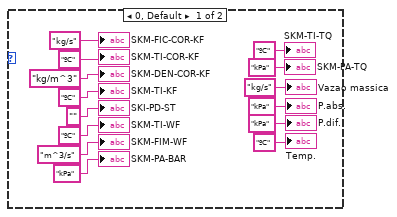
[diagram p11: hidden frame]
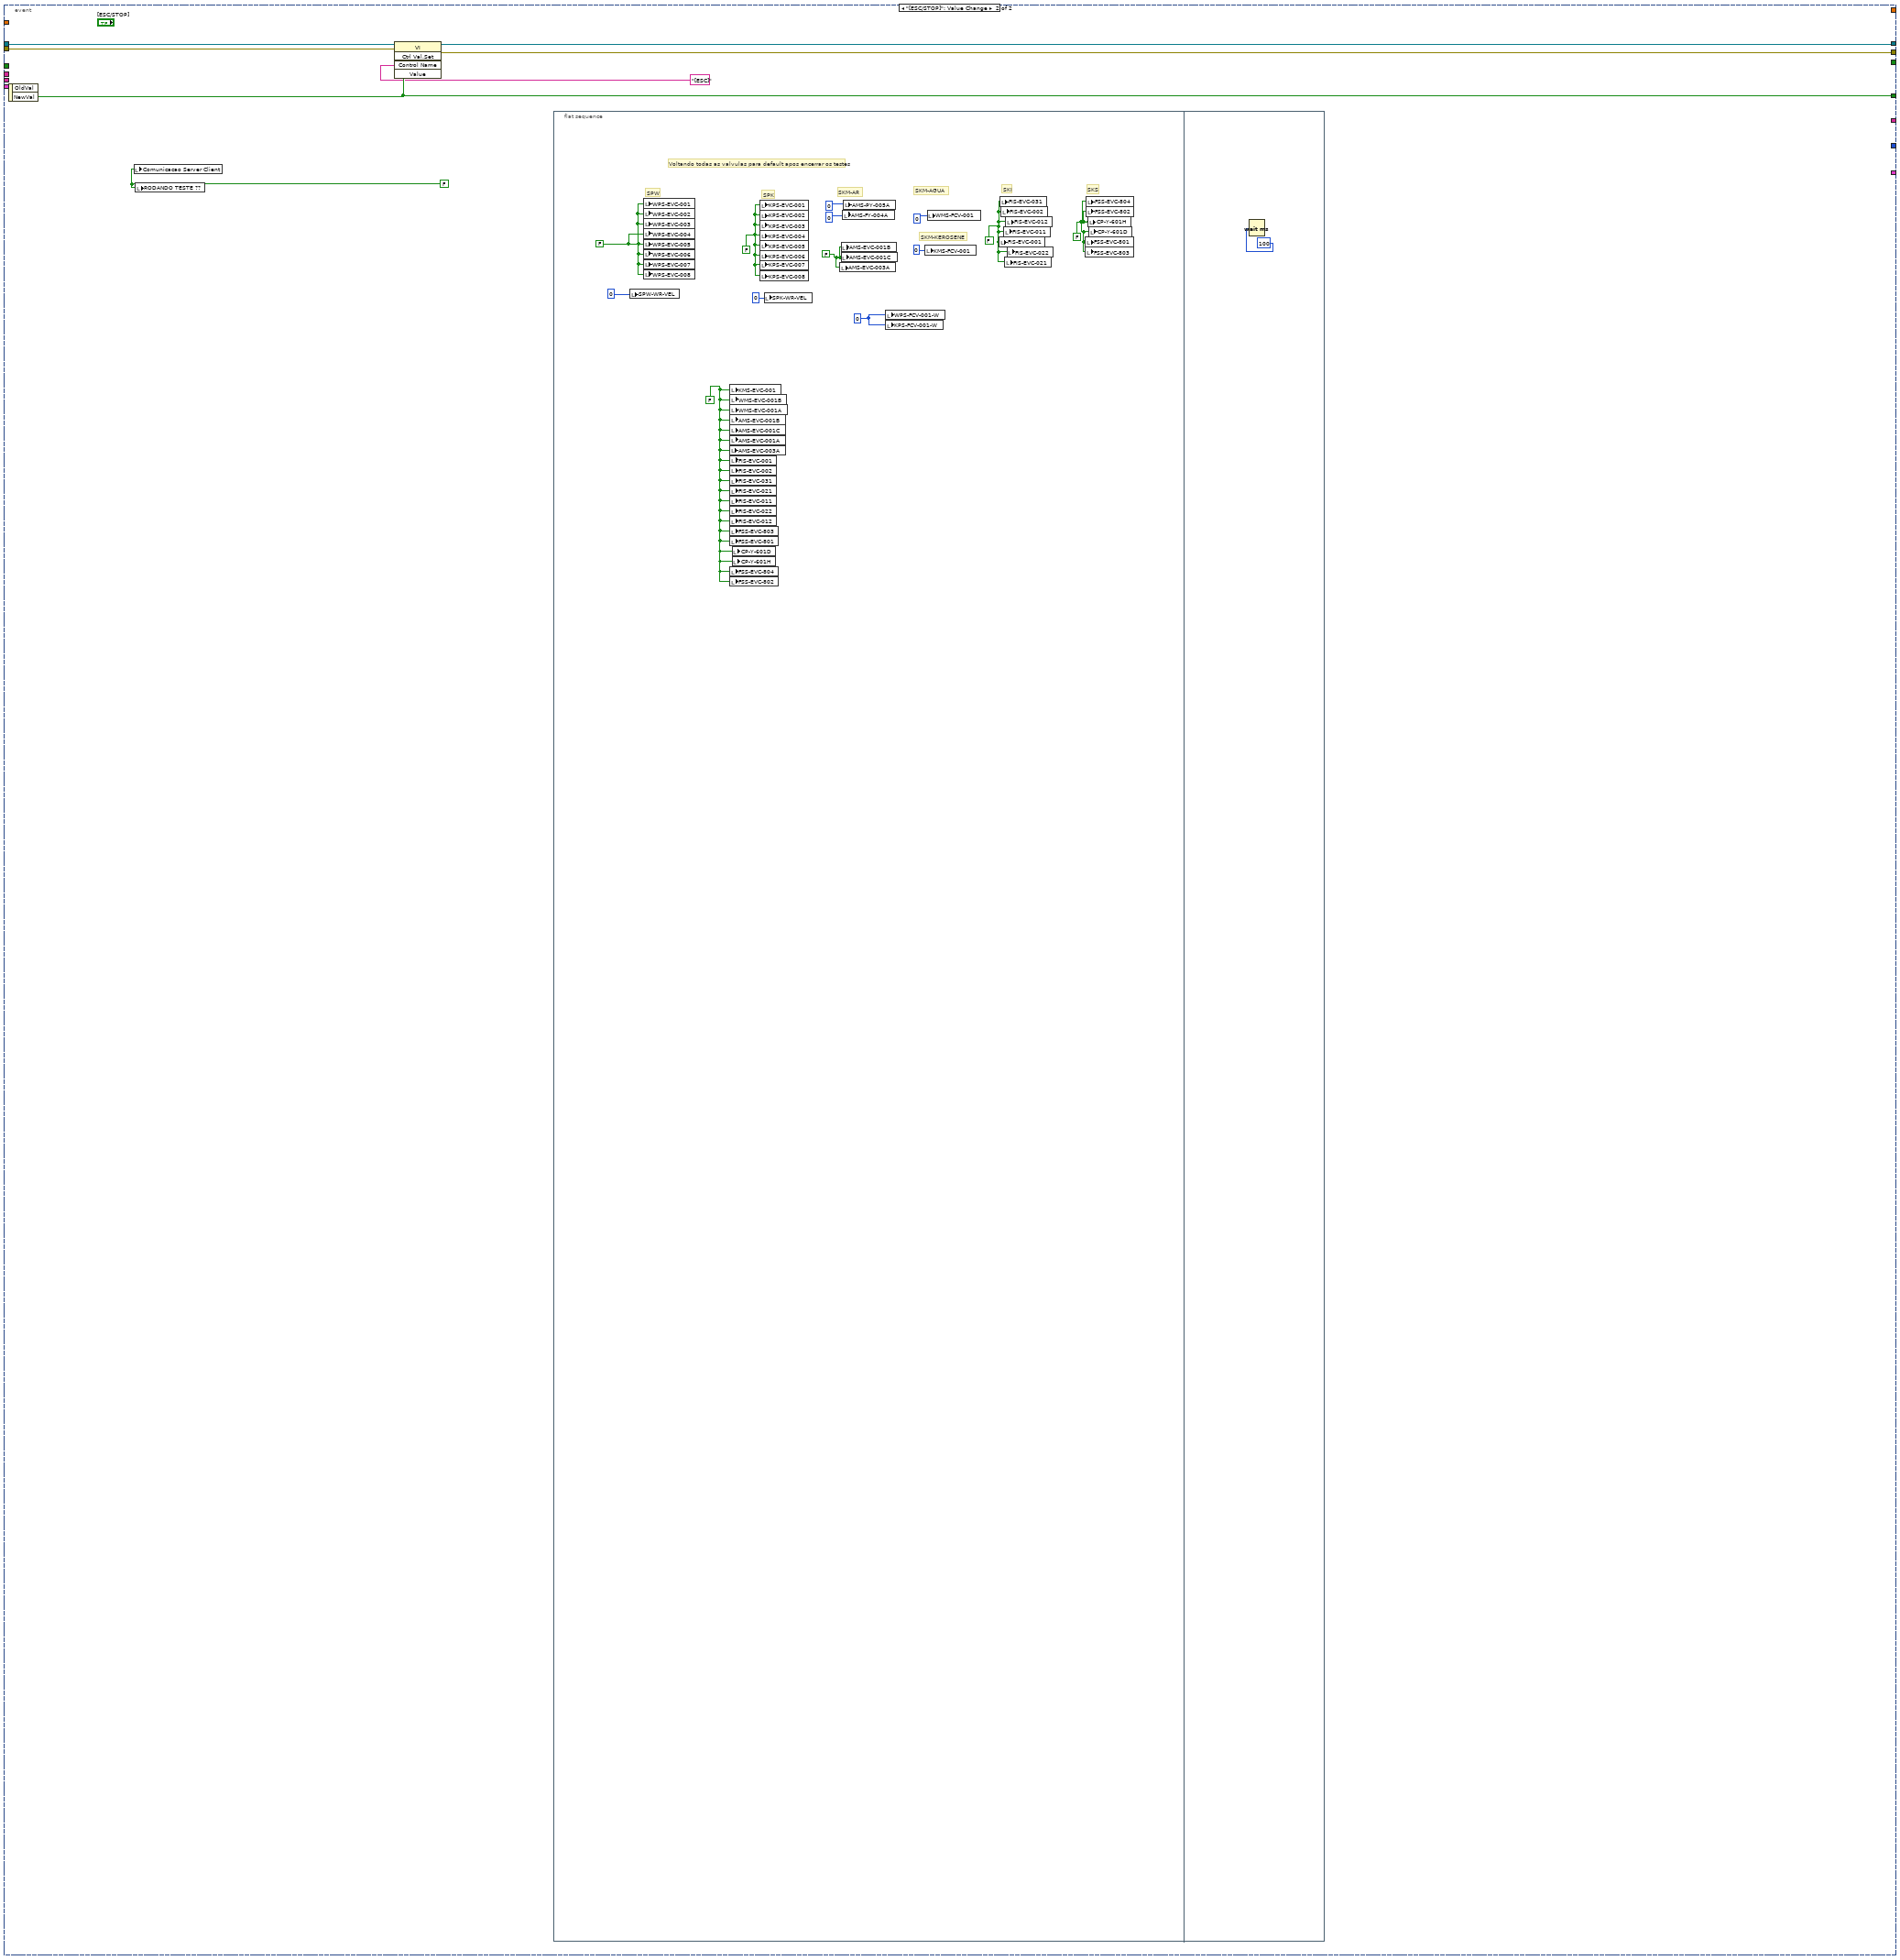
[diagram p13: hidden frame]
diagram:
  n1 = call "Run_clientSuper.vi"("Path"=path "\\\\SERVERPC\\outros/Aplicacao_Super/main_super.vi" ("path 2")) -> ("error out"=w8:errorcluster, "vi reference"=w6:refnum<vi>)  [unwired: 9 in]
  n2 = flat-sequence {
    tunnel: w8 -> [w12]
    tunnel: [w12] -> w7
    tunnel: w6 -> [w11]
    tunnel: [w11] -> w5
    tunnel: w7 -> [w19]
    tunnel: w5 -> [w18]
    tunnel: [w15] -> w4
    tunnel: [w14] -> w3
    frame #0 {
      n3 = Wait (ms)(milliseconds to wait=u32 100) -> ()  [unwired: 1 out]
    }
    frame #1 {
      n4 = call "Bloco_leiturasSuper.vi"("error in (no error)"=w19, "reference"=w18) -> ("error out"=w14:errorcluster, "reference out"=w15:refnum<vi>, "Array_Tags/Config"=w16:string[])  [unwired: 4 in, 3 out]
      n5 = call "ArrayPadraoSuper.vi"("VI"=path "\\\\SERVERPC\\outros/Aplicacao_Super/main_super.vi" ("path 2"), "Array_TAGS/Config"=w16) -> ()  [unwired: 2 in]
    }
  }
  n6 = call <vilib>:"High Resolution Relative Seconds.vi"() -> ("relative seconds"=w9:dbl)
  n7 = while {
    shift-right: [w28] -> w2
    shift-left: w4 -> [w33]
    shift-right: [w27] -> w10
    shift-left: w3 -> [w32]
    shift-right: [w21] -> _
    shift-left: w9 -> [w20]
    stop <- w36 stop-if-true
    n8 = local read "RODANDO TESTE ??"() -> (w24:bool)
    n9 = call "Bloco_leiturasSuper.vi"("error in (no error)"=w32, "reference"=w33) -> ("Status_Comunicacao"=w35:string, "Led_status"=w34:bool, "error out"=w30:errorcluster, "reference out"=w31:refnum<vi>, "Array_Tags/Config"=w29:string[], "todos_os_dados_ENTRADA"=w26:T11)  [unwired: 4 in]
    n10 = Unbundle By Name(w26) -> ("UCM.004.EEL.0200_ENTRADA.DIGITAL.CLP-601-ON"=w23:bool, "UCM.004.EEL.0300_ENTRADA.DIGITAL.CLP-ON"=w25:bool)
    n11 = Or(x=w23, y=w24) -> (x .or. y?=w22:bool)
    n12 = case shown="True" w22 {
      tunnel: [w38 w58] -> w36
      tunnel: w35 -> [_ w57]
      tunnel: w34 -> [_ w56]
      tunnel: w31 -> [w44 w55]
      tunnel: w30 -> [w43 w54]
      tunnel: w29 -> [_ w53]
      tunnel: w26 -> [_ w52]
      tunnel: [w44 w51] -> w28
      tunnel: [w43 w50] -> w27
      tunnel: w25 -> [_ w45]
      tunnel: w20 -> [w37 w47]
      tunnel: [w37 w46] -> w21
      frame False {
        n13 = Two Button Dialog(message="CLP's do 6° e 8° Andar DESLIGADOS !!! Por favor, ligue-os para continuar. ", 1:"OK" ("button name (\"OK\")"), 2:"Apenas para testes com CLP desligado !" ("T button name (\"OK\")")) -> (T button?=w39:bool)
        n14 = local write "RODANDO TESTE ??"(w39) -> ()
        n15 = Not(x=w39) -> (.not. x?=w38:bool)
      }
      frame True {
        # "CLP 6° Andar ligado ??"
        n16 = local read "RODANDO TESTE ??"() -> (w49:bool)
        n17 = Or(x=w45, y=w49) -> (x .or. y?=w48:bool)
        n18 = case shown="True" w48 {
          tunnel: [w60 w84] -> w58
          tunnel: w57 -> [_ w82]
          tunnel: w56 -> [_ w81]
          tunnel: w55 -> [w66 w80]
          tunnel: w54 -> [w65 w79]
          tunnel: w53 -> [_ w78]
          tunnel: w52 -> [_ w77]
          tunnel: [w66 w73] -> w51
          tunnel: [w65 w72] -> w50
          tunnel: w47 -> [w59 w68]
          tunnel: [w59 w67] -> w46
          frame False {
            n19 = Two Button Dialog(message="CLP do Térreo DESLIGADO !!! Por favor, ligue-o para continuar. ", 1:"OK" ("button name (\"OK\")"), 2:"Apenas para testes com CLP desligado !!" ("T button name (\"OK\")")) -> (T button?=w61:bool)
            "RODANDO TESTE ??" <- w61
            n20 = Not(x=w61) -> (.not. x?=w60:bool)
          }
          frame True {
            # "CLP Térreo ligado ??"
            n21 = event shown="[0] Timeout" {
              selector: _ -> [_ _]
              dyn-events: _ -> [_ _]
              timeout: 0 -> [_ _]
              tunnel: [_ w577] -> w84
              tunnel: w80 -> [w87 w580]
              tunnel: w79 -> [w504 w579]
              tunnel: [w504 w578] -> w71
              tunnel: w82 -> [w508 _]
              tunnel: w81 -> [w507 _]
              tunnel: w78 -> [_ _]
              tunnel: w77 -> [w88 _]
              tunnel: [w506 _] -> w70
              tunnel: [w503 _] -> w76
              tunnel: ["Abrir Editor Prioridade" _] -> w75
              tunnel: [w87 w575] -> w74
              tunnel: [w198 _] -> w69
              tunnel: w68 -> [w207 _]
              tunnel: [w206 _] -> w67
              event Timeout {
                w256 = T3 {"UCM.004.EEL.0300_SAIDA"={"DIGITAL"={"KPS-EVC-001"=FALSE, "KPS-EVC-002"=FALSE, "KPS-EVC-003"=FALSE, "KPS-EVC-004"=FALSE, "KPS-EVC-005"=FALSE, "KPS-EVC-006"=FALSE, "KPS-EVC-007"=FALSE, "KPS-EVC-008"=FALSE, "WPS-EVC-001"=FALSE, "WPS-EVC-002"=FALSE, "WPS-EVC-003"=FALSE, "WPS-EVC-004"=FALSE, "WPS-EVC-005"=FALSE, "WPS-EVC-006"=FALSE, "WPS-EVC-007"=FALSE, "WPS-EVC-008"=FALSE, "AMS-EVC-001B"=FALSE, "AMS-EVC-003A"=FALSE, "FIS-EVC-031"=FALSE, "FIS-EVC-011"=FALSE, "FIS-EVC-012"=FALSE, "FIS-EVC-021"=FALSE, "FIS-EVC-022"=FALSE, "FIS-EVC-001"=FALSE, "FIS-EVC-002"=FALSE, "KMS-EVC-001"=FALSE, "WMS-EVC-001A"=FALSE, "WMS-EVC-001B"=FALSE, "AMS-EVC-001C"=FALSE, "DG-EVC-001"=FALSE, "DG-EVC-ALL"=FALSE, "PID-PC-TQ-ON"=FALSE, "PID-FC-AR-ON"=FALSE, "PID-WF-ON"=FALSE, "PID-KF-ON"=FALSE, "PID-SA-WF-INV"=FALSE, "PID-SA-KF-INV"=FALSE, "PID-SA-AR-COR"=FALSE, "KPS-WR-ON"=FALSE, "WPS-WR-ON"=FALSE, "KPS-WR-OFF"=FALSE, "WPS-WR-OFF"=FALSE, "AMS-EVC-001A"=FALSE}, "ANALOGICO"={"AMS-PY-005A"=0, "AMS-FY-004A"=0, "WMS-FCV-001"=0, "KMS-FCV-001"=0, "X33 5"=0, "X33 6"=0, "X33 7"=0, "X33 8"=0, "X33 9"=0, "X33 10"=0, "X33 11"=0, "X33 12"=0, "X33 13"=0, "X33 14"=0, "PID-PC-TQ-SP"=0, "PID-FC-AR-SP"=0, "PID-FC-WF-SP"=0, "PID-FC-KF-SP"=0, "PID-INC-WF-SP"=0, "PID-INC-KF-SP"=0, "SPK-WR-VEL"=0, "SPW-WR-VEL"=0, "SKM-FIC-COR-KF-MAX"=0.0, "SKM-FIC-COR-KF-MIN"=0.0, "SKM-FIC-COR-WF-MAX"=0.0, "SKM-FIC-COR-WF-MIN"=0.0, "PID-PC-TQ-GP"=0.0, "PID-PC-TQ-GI"=0.0, "PID-PC-TQ-GD"=0.0, "PID-FC-AR-GP"=0.0, "PID-FC-AR-GI"=0.0, "PID-FC-AR-GD"=0.0, "PID-FC-WF-GP"=0.0, "PID-FC-WF-GI"=0.0, "PID-FC-WF-GD"=0.0, "PID-FC-KF-GP"=0.0, "PID-FC-KF-GI"=0.0, "PID-FC-KF-GD"=0.0, "PID-INV-WF-GP"=0.0, "PID-INV-WF-GI"=0.0, "PID-INV-WF-GD"=0.0, "PID-INV-KF-GP"=0.0, "PID-INV-KF-GI"=0.0, "PID-INV-KF-GD"=0.0}}, "UCM.004.EEL.0200_SAIDA"={"DIGITAL"={"FSS-EVC-801"=FALSE, "FSS-EVC-802"=FALSE, "FSS-EVC-803"=FALSE, "CP-Y-601D"=FALSE, "CP-Y-601H"=FALSE, "FSS-EVC-804"=FALSE, "SHD-CV-HD"=FALSE, "SHD-CV-ALV"=FALSE, "SHD-ON-OFF"=FALSE, "FSS-EVC-805"=FALSE, "FSS-EVC-806"=FALSE, "X31-12"=FALSE, "X31-13"=FALSE, "X31-14"=FALSE, "X31-15"=FALSE, "X31-16"=FALSE}, "ANALOGICO"={"DG-FCV-801"=0, "X33-2"=0, "FRAM-1100"=0}}, "INTERNO"={"DIGITAL"={"ITN-SI-SS-1"=FALSE, "ITN-SI-SS-2"=FALSE, "ITN-SI-SS-3"=FALSE, "ITN-SS-SW-1"=FALSE, "ITN-SS-SK-1"=FALSE, "ITN-SPW-SKM"=FALSE, "ITN-SKMW-SI"=FALSE, "ITN-SKMK-SI"=FALSE, "ITN-SKMA-SI"=FALSE, "ITN-SPK-SKM"=FALSE, "Aplicação apenas de Leitura ??"=FALSE, "SALVAR/AQUISITAR"=FALSE}, "ANALOGICO"={"ITN_Vazao_Massica_Ar"=[], "ITN_Vazao_Volumetrica_WF"=[], "ITN_Vazao_Massica_KF"=[], "ITN_Vazao_Massica_WF"=[], "ITN_Vazao_Volumetrica_KF"=[], "ITN_Temperatura"=[], "ITN_Pressão_Absoluta"=[], "ITN_Pressão_Diferencial"=[]}, "ALARMES-INTERNOS"={"ALR-AMS-001A+B"=FALSE, "ALR-AMS-001A+C"=FALSE, "ALR-AMS-001B+C"=FALSE, "ALR-AMS-001A+B+C"=FALSE, "ALR-WMS-001A+B"=FALSE}}, "ADAM_SAIDA"={"DIGITAL"={"KPS-FCV-001-W"=0.0, "WPS-FCV-001-W"=0.0, "ADAM-4024-W-2"=0.0, "ADAM-4024-W-3"=0.0}}}  # todos_os_dados_SAIDA (Controle)
                # "KMS-TIT-003? Nao deveria ser\nAMS-TIT-003? Esta no skid de medicao de ar"
                # "AMS-EVC-001E"
                # "WMS-FIT-001A = Coriolis"
                # "KMS-TIT-001"
                # "KPS-PD-001"
                # "WPS-PD-001"
                # "SKM-FIM-WF seria WMS-FIT-001B"
                # "Logica para Disabled e Enabled"
                # "Caixas de texto que indicam a unidade das medições no tipo de dado engenharia"
                # "SEPARACAO"
                # "SEPARACAO"
                # "Pump Water"
                # "Pump Kerosene"
                # "Measuring"
                # "Injection"
                # "Pump Kerosene"
                # "Pump Water"
                # "Measuring"
                # "Injection"
                n22 = event-data() -> ()  [unwired: 1 in, 3 out]
                n23 = disable-structure shown="Disabled" {
                  frame Disabled {
                    n24 = local read "WPS-FCV-001-W"() -> (w511:i16)
                    n25 = Equal?(x=w511, y=i16 0) -> (x = y?=w509:bool)
                    n26 = case shown="True" w509 {
                      frame False {
                        n27 = local read "SPW-WR-VEL"() -> (w514:i32)
                        n28 = Greater?(x=w514, y=10) -> (0:w512:bool)
                        n29 = case shown="True" w512 {
                          frame False {
                          }
                          frame True {
                            n30 = local write "WPS-EVC-001"(FALSE ("WPS-EVC-001")) -> ()
                          }
                        }
                      }
                      frame True {
                        # "Valvula fechada"
                        n31 = local read "SPW-WR-VEL"() -> (w518:i32)
                        n32 = Greater?(x=w518, y=10) -> (0:w516:bool)
                        n33 = case shown="True" w516 {
                          frame False {
                          }
                          frame True {
                            n34 = local write "SPW-WR-VEL"(10 ("SPW-WR-VEL")) -> ()
                            n35 = local write "WPS-EVC-001"(TRUE ("WPS-EVC-001")) -> ()
                          }
                        }
                      }
                    }
                  }
                  frame Enabled {
                  }
                }
                n36 = call <vilib>:"High Resolution Relative Seconds.vi"() -> ("relative seconds"=w206:dbl)
                n37 = Subtract(x=w206, y=w207) -> (x-y=→"tempo-super":dbl)
                n38 = Bundle By Name(cluster=T9 {"File Path Control"=path "", "certificado_SPK-PD-P"=FALSE, "TD-SPK-RD-VEL"=FALSE, "TD-SPK-RD-IA"=FALSE, "TD-SPK-RD-CRT"=FALSE, "TD-SPK-RD-TU"=FALSE, "TD-SPK-PD-P"=FALSE, "TD-SPK-RD-ST"=FALSE} ("Cluster_usuario_entrada_K"), "File Path Control"=path "\\\\SERVERPC\\outros/Aplicacao_Super/main_super.vi" ("path 2"), "certificado_SPK-PD-P"="certificado_SPK-PD-P", "TD-SPK-RD-VEL"="TD-SPK-RD-VEL") -> (w413:T9)
                n39 = Divide(x="WPS-FCV-001-W", y=i16 10) -> (x/y=w138:dbl)
                n40 = Bundle By Name(cluster=T8 {"VI USUARIO"=path "", "certificado_SKM-PC-TQ"=FALSE, "certificado_SKM-CV-COR"=FALSE, "certificado_SKM-CV-LAM"=FALSE, "certificado_SKM-CV-JMP"=FALSE, "certificado_SKM-FC-KF"=FALSE, "certificado_SKM-FIC-COR-KF "=FALSE, "certificado_SKM-FC-WF"=FALSE, "certificado_SKM-FIM-WF"=FALSE, "certificado_SKM-TI-KF"=FALSE, "certificado_SKM-TI-WF"=FALSE, "TD-SKM-TI-COR-AR"=FALSE, "TD-SKM-FIC-COR-AR"=FALSE, "TD-SKM-DEN-COR-AR"=FALSE, "TD-SKM-TI-LAM"=FALSE, "TD-SKM-FIC-COR-KF"=FALSE, "TD-SKM-PA-LAM"=FALSE, "TD-SKM-TI-COR-KF"=FALSE, "TD-SKM-PD-LAM"=FALSE, "TD-SKM-DEN-COR-KF"=FALSE, "certificado_SKM-PA-LAM"=FALSE, "certificado_SKM-PD-LAM"=FALSE, "certificado_SKM-TI-LAM"=FALSE, "certificado_SKM-FIC-COR-AR"=FALSE, "certificado_SKM-PA-BAR"=FALSE} ("Cluster_usuario_entrada"), "VI USUARIO"=path "\\\\SERVERPC\\outros/Aplicacao_Super/main_super.vi" ("path 2"), "TD-SKM-TI-COR-AR"="TD-SKM-TI-COR-AR", "TD-SKM-FIC-COR-AR"="TD-SKM-FIC-COR-AR", "TD-SKM-DEN-COR-AR"="TD-SKM-DEN-COR-AR", "TD-SKM-TI-LAM"="TD-SKM-TI-LAM", "TD-SKM-FIC-COR-KF"="TD-SKM-FIC-COR-KF", "TD-SKM-PA-LAM"="TD-SKM-PA-LAM", "TD-SKM-TI-COR-KF"="TD-SKM-TI-COR-KF", "TD-SKM-PD-LAM"="TD-SKM-PD-LAM", "TD-SKM-DEN-COR-KF"="TD-SKM-DEN-COR-KF") -> (w346:T8)
                n41 = Bundle By Name(cluster=T1 {"VI USUARIO"=path "", "Tipo de Dado_C"=0, "Certificado"=FALSE} ("Cluster de usuario_entrada"), "VI USUARIO"=path "\\\\SERVERPC\\outros/Aplicacao_Super/main_super.vi" ("path 2")) -> (w297:T1)
                n42 = Divide(x="KPS-FCV-001-W", y=i16 10) -> (x/y=w139:dbl)
                n43 = Bundle By Name(cluster=T3 {"UCM.004.EEL.0300_SAIDA"={"DIGITAL"={"KPS-EVC-001"=FALSE, "KPS-EVC-002"=FALSE, "KPS-EVC-003"=FALSE, "KPS-EVC-004"=FALSE, "KPS-EVC-005"=FALSE, "KPS-EVC-006"=FALSE, "KPS-EVC-007"=FALSE, "KPS-EVC-008"=FALSE, "WPS-EVC-001"=FALSE, "WPS-EVC-002"=FALSE, "WPS-EVC-003"=FALSE, "WPS-EVC-004"=FALSE, "WPS-EVC-005"=FALSE, "WPS-EVC-006"=FALSE, "WPS-EVC-007"=FALSE, "WPS-EVC-008"=FALSE, "AMS-EVC-001B"=FALSE, "AMS-EVC-003A"=FALSE, "FIS-EVC-031"=FALSE, "FIS-EVC-011"=FALSE, "FIS-EVC-012"=FALSE, "FIS-EVC-021"=FALSE, "FIS-EVC-022"=FALSE, "FIS-EVC-001"=FALSE, "FIS-EVC-002"=FALSE, "KMS-EVC-001"=FALSE, "WMS-EVC-001A"=FALSE, "WMS-EVC-001B"=FALSE, "AMS-EVC-001C"=FALSE, "DG-EVC-001"=FALSE, "DG-EVC-ALL"=FALSE, "PID-PC-TQ-ON"=FALSE, "PID-FC-AR-ON"=FALSE, "PID-WF-ON"=FALSE, "PID-KF-ON"=FALSE, "PID-SA-WF-INV"=FALSE, "PID-SA-KF-INV"=FALSE, "PID-SA-AR-COR"=FALSE, "KPS-WR-ON"=FALSE, "WPS-WR-ON"=FALSE, "KPS-WR-OFF"=FALSE, "WPS-WR-OFF"=FALSE, "AMS-EVC-001A"=FALSE}, "ANALOGICO"={"AMS-PY-005A"=0, "AMS-FY-004A"=0, "WMS-FCV-001"=0, "KMS-FCV-001"=0, "X33 5"=0, "X33 6"=0, "X33 7"=0, "X33 8"=0, "X33 9"=0, "X33 10"=0, "X33 11"=0, "X33 12"=0, "X33 13"=0, "X33 14"=0, "PID-PC-TQ-SP"=0, "PID-FC-AR-SP"=0, "PID-FC-WF-SP"=0, "PID-FC-KF-SP"=0, "PID-INC-WF-SP"=0, "PID-INC-KF-SP"=0, "SPK-WR-VEL"=0, "SPW-WR-VEL"=0, "SKM-FIC-COR-KF-MAX"=0.0, "SKM-FIC-COR-KF-MIN"=0.0, "SKM-FIC-COR-WF-MAX"=0.0, "SKM-FIC-COR-WF-MIN"=0.0, "PID-PC-TQ-GP"=0.0, "PID-PC-TQ-GI"=0.0, "PID-PC-TQ-GD"=0.0, "PID-FC-AR-GP"=0.0, "PID-FC-AR-GI"=0.0, "PID-FC-AR-GD"=0.0, "PID-FC-WF-GP"=0.0, "PID-FC-WF-GI"=0.0, "PID-FC-WF-GD"=0.0, "PID-FC-KF-GP"=0.0, "PID-FC-KF-GI"=0.0, "PID-FC-KF-GD"=0.0, "PID-INV-WF-GP"=0.0, "PID-INV-WF-GI"=0.0, "PID-INV-WF-GD"=0.0, "PID-INV-KF-GP"=0.0, "PID-INV-KF-GI"=0.0, "PID-INV-KF-GD"=0.0}}, "UCM.004.EEL.0200_SAIDA"={"DIGITAL"={"FSS-EVC-801"=FALSE, "FSS-EVC-802"=FALSE, "FSS-EVC-803"=FALSE, "CP-Y-601D"=FALSE, "CP-Y-601H"=FALSE, "FSS-EVC-804"=FALSE, "SHD-CV-HD"=FALSE, "SHD-CV-ALV"=FALSE, "SHD-ON-OFF"=FALSE, "FSS-EVC-805"=FALSE, "FSS-EVC-806"=FALSE, "X31-12"=FALSE, "X31-13"=FALSE, "X31-14"=FALSE, "X31-15"=FALSE, "X31-16"=FALSE}, "ANALOGICO"={"DG-FCV-801"=0, "X33-2"=0, "FRAM-1100"=0}}, "INTERNO"={"DIGITAL"={"ITN-SI-SS-1"=FALSE, "ITN-SI-SS-2"=FALSE, "ITN-SI-SS-3"=FALSE, "ITN-SS-SW-1"=FALSE, "ITN-SS-SK-1"=FALSE, "ITN-SPW-SKM"=FALSE, "ITN-SKMW-SI"=FALSE, "ITN-SKMK-SI"=FALSE, "ITN-SKMA-SI"=FALSE, "ITN-SPK-SKM"=FALSE, "Aplicação apenas de Leitura ??"=FALSE, "SALVAR/AQUISITAR"=FALSE}, "ANALOGICO"={"ITN_Vazao_Massica_Ar"=[], "ITN_Vazao_Volumetrica_WF"=[], "ITN_Vazao_Massica_KF"=[], "ITN_Vazao_Massica_WF"=[], "ITN_Vazao_Volumetrica_KF"=[], "ITN_Temperatura"=[], "ITN_Pressão_Absoluta"=[], "ITN_Pressão_Diferencial"=[]}, "ALARMES-INTERNOS"={"ALR-AMS-001A+B"=FALSE, "ALR-AMS-001A+C"=FALSE, "ALR-AMS-001B+C"=FALSE, "ALR-AMS-001A+B+C"=FALSE, "ALR-WMS-001A+B"=FALSE}}, "ADAM_SAIDA"={"DIGITAL"={"KPS-FCV-001-W"=0.0, "WPS-FCV-001-W"=0.0, "ADAM-4024-W-2"=0.0, "ADAM-4024-W-3"=0.0}}} ("todos_os_dados_SAIDA"), "UCM.004.EEL.0300_SAIDA.DIGITAL.WPS-EVC-001"="WPS-EVC-001", "UCM.004.EEL.0300_SAIDA.DIGITAL.WPS-EVC-002"="WPS-EVC-002", "UCM.004.EEL.0300_SAIDA.DIGITAL.WPS-EVC-003"="WPS-EVC-003", "UCM.004.EEL.0300_SAIDA.DIGITAL.WPS-EVC-004"="WPS-EVC-004", "UCM.004.EEL.0300_SAIDA.DIGITAL.WPS-EVC-005"="WPS-EVC-005", "UCM.004.EEL.0300_SAIDA.DIGITAL.WPS-EVC-006"="WPS-EVC-006", "UCM.004.EEL.0300_SAIDA.DIGITAL.WPS-EVC-007"="WPS-EVC-007", "UCM.004.EEL.0300_SAIDA.DIGITAL.WPS-EVC-008"="WPS-EVC-008", "UCM.004.EEL.0300_SAIDA.DIGITAL.PID-WF-ON"="PID-WF-ON", "UCM.004.EEL.0300_SAIDA.DIGITAL.WPS-WR-ON"="WPS-WR-ON", "UCM.004.EEL.0300_SAIDA.DIGITAL.WPS-WR-OFF"="WPS-WR-OFF", "UCM.004.EEL.0300_SAIDA.ANALOGICO.SPW-WR-VEL"="SPW-WR-VEL", "ADAM_SAIDA.DIGITAL.WPS-FCV-001-W"=w138) -> (w501:T3)
                n44 = Bundle By Name(cluster=T10 {"Path Main"=path "", "certificado_SPW-PD-P"=FALSE, "TD-SPW-RD-VEL"=FALSE, "TD-SPW-RD-IA"=FALSE, "TD-SPW-RD-CRT"=FALSE, "TD-SPW-RD-TU"=FALSE, "TD-SPW-PD-P"=FALSE, "TD-SPW-RD-ST"=FALSE} ("Cluster_usuario_entrada"), "Path Main"=path "\\\\SERVERPC\\outros/Aplicacao_Super/main_super.vi" ("path 2"), "certificado_SPW-PD-P"="certificado_SPW-PD-P", "TD-SPW-RD-VEL"="TD-SPW-RD-VEL") -> (w199:T10)
                n45 = Bundle By Name(cluster=T3 {"UCM.004.EEL.0300_SAIDA"={"DIGITAL"={"KPS-EVC-001"=FALSE, "KPS-EVC-002"=FALSE, "KPS-EVC-003"=FALSE, "KPS-EVC-004"=FALSE, "KPS-EVC-005"=FALSE, "KPS-EVC-006"=FALSE, "KPS-EVC-007"=FALSE, "KPS-EVC-008"=FALSE, "WPS-EVC-001"=FALSE, "WPS-EVC-002"=FALSE, "WPS-EVC-003"=FALSE, "WPS-EVC-004"=FALSE, "WPS-EVC-005"=FALSE, "WPS-EVC-006"=FALSE, "WPS-EVC-007"=FALSE, "WPS-EVC-008"=FALSE, "AMS-EVC-001B"=FALSE, "AMS-EVC-003A"=FALSE, "FIS-EVC-031"=FALSE, "FIS-EVC-011"=FALSE, "FIS-EVC-012"=FALSE, "FIS-EVC-021"=FALSE, "FIS-EVC-022"=FALSE, "FIS-EVC-001"=FALSE, "FIS-EVC-002"=FALSE, "KMS-EVC-001"=FALSE, "WMS-EVC-001A"=FALSE, "WMS-EVC-001B"=FALSE, "AMS-EVC-001C"=FALSE, "DG-EVC-001"=FALSE, "DG-EVC-ALL"=FALSE, "PID-PC-TQ-ON"=FALSE, "PID-FC-AR-ON"=FALSE, "PID-WF-ON"=FALSE, "PID-KF-ON"=FALSE, "PID-SA-WF-INV"=FALSE, "PID-SA-KF-INV"=FALSE, "PID-SA-AR-COR"=FALSE, "KPS-WR-ON"=FALSE, "WPS-WR-ON"=FALSE, "KPS-WR-OFF"=FALSE, "WPS-WR-OFF"=FALSE, "AMS-EVC-001A"=FALSE}, "ANALOGICO"={"AMS-PY-005A"=0, "AMS-FY-004A"=0, "WMS-FCV-001"=0, "KMS-FCV-001"=0, "X33 5"=0, "X33 6"=0, "X33 7"=0, "X33 8"=0, "X33 9"=0, "X33 10"=0, "X33 11"=0, "X33 12"=0, "X33 13"=0, "X33 14"=0, "PID-PC-TQ-SP"=0, "PID-FC-AR-SP"=0, "PID-FC-WF-SP"=0, "PID-FC-KF-SP"=0, "PID-INC-WF-SP"=0, "PID-INC-KF-SP"=0, "SPK-WR-VEL"=0, "SPW-WR-VEL"=0, "SKM-FIC-COR-KF-MAX"=0.0, "SKM-FIC-COR-KF-MIN"=0.0, "SKM-FIC-COR-WF-MAX"=0.0, "SKM-FIC-COR-WF-MIN"=0.0, "PID-PC-TQ-GP"=0.0, "PID-PC-TQ-GI"=0.0, "PID-PC-TQ-GD"=0.0, "PID-FC-AR-GP"=0.0, "PID-FC-AR-GI"=0.0, "PID-FC-AR-GD"=0.0, "PID-FC-WF-GP"=0.0, "PID-FC-WF-GI"=0.0, "PID-FC-WF-GD"=0.0, "PID-FC-KF-GP"=0.0, "PID-FC-KF-GI"=0.0, "PID-FC-KF-GD"=0.0, "PID-INV-WF-GP"=0.0, "PID-INV-WF-GI"=0.0, "PID-INV-WF-GD"=0.0, "PID-INV-KF-GP"=0.0, "PID-INV-KF-GI"=0.0, "PID-INV-KF-GD"=0.0}}, "UCM.004.EEL.0200_SAIDA"={"DIGITAL"={"FSS-EVC-801"=FALSE, "FSS-EVC-802"=FALSE, "FSS-EVC-803"=FALSE, "CP-Y-601D"=FALSE, "CP-Y-601H"=FALSE, "FSS-EVC-804"=FALSE, "SHD-CV-HD"=FALSE, "SHD-CV-ALV"=FALSE, "SHD-ON-OFF"=FALSE, "FSS-EVC-805"=FALSE, "FSS-EVC-806"=FALSE, "X31-12"=FALSE, "X31-13"=FALSE, "X31-14"=FALSE, "X31-15"=FALSE, "X31-16"=FALSE}, "ANALOGICO"={"DG-FCV-801"=0, "X33-2"=0, "FRAM-1100"=0}}, "INTERNO"={"DIGITAL"={"ITN-SI-SS-1"=FALSE, "ITN-SI-SS-2"=FALSE, "ITN-SI-SS-3"=FALSE, "ITN-SS-SW-1"=FALSE, "ITN-SS-SK-1"=FALSE, "ITN-SPW-SKM"=FALSE, "ITN-SKMW-SI"=FALSE, "ITN-SKMK-SI"=FALSE, "ITN-SKMA-SI"=FALSE, "ITN-SPK-SKM"=FALSE, "Aplicação apenas de Leitura ??"=FALSE, "SALVAR/AQUISITAR"=FALSE}, "ANALOGICO"={"ITN_Vazao_Massica_Ar"=[], "ITN_Vazao_Volumetrica_WF"=[], "ITN_Vazao_Massica_KF"=[], "ITN_Vazao_Massica_WF"=[], "ITN_Vazao_Volumetrica_KF"=[], "ITN_Temperatura"=[], "ITN_Pressão_Absoluta"=[], "ITN_Pressão_Diferencial"=[]}, "ALARMES-INTERNOS"={"ALR-AMS-001A+B"=FALSE, "ALR-AMS-001A+C"=FALSE, "ALR-AMS-001B+C"=FALSE, "ALR-AMS-001A+B+C"=FALSE, "ALR-WMS-001A+B"=FALSE}}, "ADAM_SAIDA"={"DIGITAL"={"KPS-FCV-001-W"=0.0, "WPS-FCV-001-W"=0.0, "ADAM-4024-W-2"=0.0, "ADAM-4024-W-3"=0.0}}} ("todos_os_dados_SAIDA (controle)"), "ADAM_SAIDA.DIGITAL.KPS-FCV-001-W"=w139, "UCM.004.EEL.0300_SAIDA.DIGITAL.KPS-EVC-001"="KPS-EVC-001", "UCM.004.EEL.0300_SAIDA.DIGITAL.KPS-EVC-002"="KPS-EVC-002", "UCM.004.EEL.0300_SAIDA.DIGITAL.KPS-EVC-003"="KPS-EVC-003", "UCM.004.EEL.0300_SAIDA.DIGITAL.KPS-EVC-004"="KPS-EVC-004", "UCM.004.EEL.0300_SAIDA.DIGITAL.KPS-EVC-005"="KPS-EVC-005", "UCM.004.EEL.0300_SAIDA.DIGITAL.KPS-EVC-006"="KPS-EVC-006", "UCM.004.EEL.0300_SAIDA.DIGITAL.KPS-EVC-007"="KPS-EVC-007", "UCM.004.EEL.0300_SAIDA.DIGITAL.KPS-EVC-008"="KPS-EVC-008", "UCM.004.EEL.0300_SAIDA.DIGITAL.KPS-WR-ON"="KPS-WR-ON", "UCM.004.EEL.0300_SAIDA.DIGITAL.KPS-WR-OFF"="KPS-WR-OFF", "UCM.004.EEL.0300_SAIDA.DIGITAL.PID-KF-ON"="PID-KF-ON", "UCM.004.EEL.0300_SAIDA.ANALOGICO.SPK-WR-VEL"="SPK-WR-VEL") -> (w414:T3)
                n46 = Bundle By Name(cluster=T3 {"UCM.004.EEL.0300_SAIDA"={"DIGITAL"={"KPS-EVC-001"=FALSE, "KPS-EVC-002"=FALSE, "KPS-EVC-003"=FALSE, "KPS-EVC-004"=FALSE, "KPS-EVC-005"=FALSE, "KPS-EVC-006"=FALSE, "KPS-EVC-007"=FALSE, "KPS-EVC-008"=FALSE, "WPS-EVC-001"=FALSE, "WPS-EVC-002"=FALSE, "WPS-EVC-003"=FALSE, "WPS-EVC-004"=FALSE, "WPS-EVC-005"=FALSE, "WPS-EVC-006"=FALSE, "WPS-EVC-007"=FALSE, "WPS-EVC-008"=FALSE, "AMS-EVC-001B"=FALSE, "AMS-EVC-003A"=FALSE, "FIS-EVC-031"=FALSE, "FIS-EVC-011"=FALSE, "FIS-EVC-012"=FALSE, "FIS-EVC-021"=FALSE, "FIS-EVC-022"=FALSE, "FIS-EVC-001"=FALSE, "FIS-EVC-002"=FALSE, "KMS-EVC-001"=FALSE, "WMS-EVC-001A"=FALSE, "WMS-EVC-001B"=FALSE, "AMS-EVC-001C"=FALSE, "DG-EVC-001"=FALSE, "DG-EVC-ALL"=FALSE, "PID-PC-TQ-ON"=FALSE, "PID-FC-AR-ON"=FALSE, "PID-WF-ON"=FALSE, "PID-KF-ON"=FALSE, "PID-SA-WF-INV"=FALSE, "PID-SA-KF-INV"=FALSE, "PID-SA-AR-COR"=FALSE, "KPS-WR-ON"=FALSE, "WPS-WR-ON"=FALSE, "KPS-WR-OFF"=FALSE, "WPS-WR-OFF"=FALSE, "AMS-EVC-001A"=FALSE}, "ANALOGICO"={"AMS-PY-005A"=0, "AMS-FY-004A"=0, "WMS-FCV-001"=0, "KMS-FCV-001"=0, "X33 5"=0, "X33 6"=0, "X33 7"=0, "X33 8"=0, "X33 9"=0, "X33 10"=0, "X33 11"=0, "X33 12"=0, "X33 13"=0, "X33 14"=0, "PID-PC-TQ-SP"=0, "PID-FC-AR-SP"=0, "PID-FC-WF-SP"=0, "PID-FC-KF-SP"=0, "PID-INC-WF-SP"=0, "PID-INC-KF-SP"=0, "SPK-WR-VEL"=0, "SPW-WR-VEL"=0, "SKM-FIC-COR-KF-MAX"=0.0, "SKM-FIC-COR-KF-MIN"=0.0, "SKM-FIC-COR-WF-MAX"=0.0, "SKM-FIC-COR-WF-MIN"=0.0, "PID-PC-TQ-GP"=0.0, "PID-PC-TQ-GI"=0.0, "PID-PC-TQ-GD"=0.0, "PID-FC-AR-GP"=0.0, "PID-FC-AR-GI"=0.0, "PID-FC-AR-GD"=0.0, "PID-FC-WF-GP"=0.0, "PID-FC-WF-GI"=0.0, "PID-FC-WF-GD"=0.0, "PID-FC-KF-GP"=0.0, "PID-FC-KF-GI"=0.0, "PID-FC-KF-GD"=0.0, "PID-INV-WF-GP"=0.0, "PID-INV-WF-GI"=0.0, "PID-INV-WF-GD"=0.0, "PID-INV-KF-GP"=0.0, "PID-INV-KF-GI"=0.0, "PID-INV-KF-GD"=0.0}}, "UCM.004.EEL.0200_SAIDA"={"DIGITAL"={"FSS-EVC-801"=FALSE, "FSS-EVC-802"=FALSE, "FSS-EVC-803"=FALSE, "CP-Y-601D"=FALSE, "CP-Y-601H"=FALSE, "FSS-EVC-804"=FALSE, "SHD-CV-HD"=FALSE, "SHD-CV-ALV"=FALSE, "SHD-ON-OFF"=FALSE, "FSS-EVC-805"=FALSE, "FSS-EVC-806"=FALSE, "X31-12"=FALSE, "X31-13"=FALSE, "X31-14"=FALSE, "X31-15"=FALSE, "X31-16"=FALSE}, "ANALOGICO"={"DG-FCV-801"=0, "X33-2"=0, "FRAM-1100"=0}}, "INTERNO"={"DIGITAL"={"ITN-SI-SS-1"=FALSE, "ITN-SI-SS-2"=FALSE, "ITN-SI-SS-3"=FALSE, "ITN-SS-SW-1"=FALSE, "ITN-SS-SK-1"=FALSE, "ITN-SPW-SKM"=FALSE, "ITN-SKMW-SI"=FALSE, "ITN-SKMK-SI"=FALSE, "ITN-SKMA-SI"=FALSE, "ITN-SPK-SKM"=FALSE, "Aplicação apenas de Leitura ??"=FALSE, "SALVAR/AQUISITAR"=FALSE}, "ANALOGICO"={"ITN_Vazao_Massica_Ar"=[], "ITN_Vazao_Volumetrica_WF"=[], "ITN_Vazao_Massica_KF"=[], "ITN_Vazao_Massica_WF"=[], "ITN_Vazao_Volumetrica_KF"=[], "ITN_Temperatura"=[], "ITN_Pressão_Absoluta"=[], "ITN_Pressão_Diferencial"=[]}, "ALARMES-INTERNOS"={"ALR-AMS-001A+B"=FALSE, "ALR-AMS-001A+C"=FALSE, "ALR-AMS-001B+C"=FALSE, "ALR-AMS-001A+B+C"=FALSE, "ALR-WMS-001A+B"=FALSE}}, "ADAM_SAIDA"={"DIGITAL"={"KPS-FCV-001-W"=0.0, "WPS-FCV-001-W"=0.0, "ADAM-4024-W-2"=0.0, "ADAM-4024-W-3"=0.0}}} ("todos_os_dados_SAIDA_C"), "UCM.004.EEL.0300_SAIDA.DIGITAL.FIS-EVC-031"="FIS-EVC-031", "UCM.004.EEL.0300_SAIDA.DIGITAL.FIS-EVC-011"="FIS-EVC-011", "UCM.004.EEL.0300_SAIDA.DIGITAL.FIS-EVC-012"="FIS-EVC-012", "UCM.004.EEL.0300_SAIDA.DIGITAL.FIS-EVC-021"="FIS-EVC-021", "UCM.004.EEL.0300_SAIDA.DIGITAL.FIS-EVC-022"="FIS-EVC-022", "UCM.004.EEL.0300_SAIDA.DIGITAL.FIS-EVC-001"="FIS-EVC-001", "UCM.004.EEL.0300_SAIDA.DIGITAL.FIS-EVC-002"="FIS-EVC-002") -> (w321:T3)
                n47 = Bundle By Name(cluster=w256, "UCM.004.EEL.0200_SAIDA.DIGITAL.FSS-EVC-801"="FSS-EVC-801", "UCM.004.EEL.0200_SAIDA.DIGITAL.FSS-EVC-802"="FSS-EVC-802", "UCM.004.EEL.0200_SAIDA.DIGITAL.FSS-EVC-803"="FSS-EVC-803", "UCM.004.EEL.0200_SAIDA.DIGITAL.CP-Y-601D"="CP-Y-601D", "UCM.004.EEL.0200_SAIDA.DIGITAL.CP-Y-601H"="CP-Y-601H", "UCM.004.EEL.0200_SAIDA.DIGITAL.FSS-EVC-804"="FSS-EVC-804") -> (w257:T3)
                n48 = Bundle By Name(cluster=T3 {"UCM.004.EEL.0300_SAIDA"={"DIGITAL"={"KPS-EVC-001"=FALSE, "KPS-EVC-002"=FALSE, "KPS-EVC-003"=FALSE, "KPS-EVC-004"=FALSE, "KPS-EVC-005"=FALSE, "KPS-EVC-006"=FALSE, "KPS-EVC-007"=FALSE, "KPS-EVC-008"=FALSE, "WPS-EVC-001"=FALSE, "WPS-EVC-002"=FALSE, "WPS-EVC-003"=FALSE, "WPS-EVC-004"=FALSE, "WPS-EVC-005"=FALSE, "WPS-EVC-006"=FALSE, "WPS-EVC-007"=FALSE, "WPS-EVC-008"=FALSE, "AMS-EVC-001B"=FALSE, "AMS-EVC-003A"=FALSE, "FIS-EVC-031"=FALSE, "FIS-EVC-011"=FALSE, "FIS-EVC-012"=FALSE, "FIS-EVC-021"=FALSE, "FIS-EVC-022"=FALSE, "FIS-EVC-001"=FALSE, "FIS-EVC-002"=FALSE, "KMS-EVC-001"=FALSE, "WMS-EVC-001A"=FALSE, "WMS-EVC-001B"=FALSE, "AMS-EVC-001C"=FALSE, "DG-EVC-001"=FALSE, "DG-EVC-ALL"=FALSE, "PID-PC-TQ-ON"=FALSE, "PID-FC-AR-ON"=FALSE, "PID-WF-ON"=FALSE, "PID-KF-ON"=FALSE, "PID-SA-WF-INV"=FALSE, "PID-SA-KF-INV"=FALSE, "PID-SA-AR-COR"=FALSE, "KPS-WR-ON"=FALSE, "WPS-WR-ON"=FALSE, "KPS-WR-OFF"=FALSE, "WPS-WR-OFF"=FALSE, "AMS-EVC-001A"=FALSE}, "ANALOGICO"={"AMS-PY-005A"=0, "AMS-FY-004A"=0, "WMS-FCV-001"=0, "KMS-FCV-001"=0, "X33 5"=0, "X33 6"=0, "X33 7"=0, "X33 8"=0, "X33 9"=0, "X33 10"=0, "X33 11"=0, "X33 12"=0, "X33 13"=0, "X33 14"=0, "PID-PC-TQ-SP"=0, "PID-FC-AR-SP"=0, "PID-FC-WF-SP"=0, "PID-FC-KF-SP"=0, "PID-INC-WF-SP"=0, "PID-INC-KF-SP"=0, "SPK-WR-VEL"=0, "SPW-WR-VEL"=0, "SKM-FIC-COR-KF-MAX"=0.0, "SKM-FIC-COR-KF-MIN"=0.0, "SKM-FIC-COR-WF-MAX"=0.0, "SKM-FIC-COR-WF-MIN"=0.0, "PID-PC-TQ-GP"=0.0, "PID-PC-TQ-GI"=0.0, "PID-PC-TQ-GD"=0.0, "PID-FC-AR-GP"=0.0, "PID-FC-AR-GI"=0.0, "PID-FC-AR-GD"=0.0, "PID-FC-WF-GP"=0.0, "PID-FC-WF-GI"=0.0, "PID-FC-WF-GD"=0.0, "PID-FC-KF-GP"=0.0, "PID-FC-KF-GI"=0.0, "PID-FC-KF-GD"=0.0, "PID-INV-WF-GP"=0.0, "PID-INV-WF-GI"=0.0, "PID-INV-WF-GD"=0.0, "PID-INV-KF-GP"=0.0, "PID-INV-KF-GI"=0.0, "PID-INV-KF-GD"=0.0}}, "UCM.004.EEL.0200_SAIDA"={"DIGITAL"={"FSS-EVC-801"=FALSE, "FSS-EVC-802"=FALSE, "FSS-EVC-803"=FALSE, "CP-Y-601D"=FALSE, "CP-Y-601H"=FALSE, "FSS-EVC-804"=FALSE, "SHD-CV-HD"=FALSE, "SHD-CV-ALV"=FALSE, "SHD-ON-OFF"=FALSE, "FSS-EVC-805"=FALSE, "FSS-EVC-806"=FALSE, "X31-12"=FALSE, "X31-13"=FALSE, "X31-14"=FALSE, "X31-15"=FALSE, "X31-16"=FALSE}, "ANALOGICO"={"DG-FCV-801"=0, "X33-2"=0, "FRAM-1100"=0}}, "INTERNO"={"DIGITAL"={"ITN-SI-SS-1"=FALSE, "ITN-SI-SS-2"=FALSE, "ITN-SI-SS-3"=FALSE, "ITN-SS-SW-1"=FALSE, "ITN-SS-SK-1"=FALSE, "ITN-SPW-SKM"=FALSE, "ITN-SKMW-SI"=FALSE, "ITN-SKMK-SI"=FALSE, "ITN-SKMA-SI"=FALSE, "ITN-SPK-SKM"=FALSE, "Aplicação apenas de Leitura ??"=FALSE, "SALVAR/AQUISITAR"=FALSE}, "ANALOGICO"={"ITN_Vazao_Massica_Ar"=[], "ITN_Vazao_Volumetrica_WF"=[], "ITN_Vazao_Massica_KF"=[], "ITN_Vazao_Massica_WF"=[], "ITN_Vazao_Volumetrica_KF"=[], "ITN_Temperatura"=[], "ITN_Pressão_Absoluta"=[], "ITN_Pressão_Diferencial"=[]}, "ALARMES-INTERNOS"={"ALR-AMS-001A+B"=FALSE, "ALR-AMS-001A+C"=FALSE, "ALR-AMS-001B+C"=FALSE, "ALR-AMS-001A+B+C"=FALSE, "ALR-WMS-001A+B"=FALSE}}, "ADAM_SAIDA"={"DIGITAL"={"KPS-FCV-001-W"=0.0, "WPS-FCV-001-W"=0.0, "ADAM-4024-W-2"=0.0, "ADAM-4024-W-3"=0.0}}} ("todos_os_dados_SAIDA"), "UCM.004.EEL.0300_SAIDA.DIGITAL.KMS-EVC-001"="KMS-EVC-001", "UCM.004.EEL.0300_SAIDA.DIGITAL.AMS-EVC-001A"="AMS-EVC-001A", "UCM.004.EEL.0300_SAIDA.DIGITAL.WMS-EVC-001A"="WMS-EVC-001A", "UCM.004.EEL.0300_SAIDA.DIGITAL.WMS-EVC-001B"="WMS-EVC-001B", "UCM.004.EEL.0300_SAIDA.DIGITAL.AMS-EVC-001B"="AMS-EVC-001B", "UCM.004.EEL.0300_SAIDA.DIGITAL.AMS-EVC-003A"="AMS-EVC-003A", "UCM.004.EEL.0300_SAIDA.DIGITAL.AMS-EVC-001C"="AMS-EVC-001C", "UCM.004.EEL.0300_SAIDA.ANALOGICO.AMS-PY-005A"="AMS-PY-005A", "UCM.004.EEL.0300_SAIDA.ANALOGICO.AMS-FY-004A"="AMS-FY-004A", "UCM.004.EEL.0300_SAIDA.ANALOGICO.WMS-FCV-001"="WMS-FCV-001", "UCM.004.EEL.0300_SAIDA.ANALOGICO.KMS-FCV-001"="KMS-FCV-001") -> (w348:T3)
                n49 = Unbundle By Name(w88) -> ("UCM.004.EEL.0300_ENTRADA.DIGITAL.AMS-ZT-001A"=w94:bool, "UCM.004.EEL.0300_ENTRADA.DIGITAL.AMS-ZT-001B"=w93:bool, "UCM.004.EEL.0300_ENTRADA.DIGITAL.AMS-ZT-001C"=w92:bool)
                n50 = Unbundle By Name(w88) -> ()  [unwired: 2 out]
                n51 = Not(x=w94) -> (.not. x?=w89:bool)
                n52 = Not(x=w93) -> (.not. x?=w90:bool)
                n53 = Not(x=w92) -> (.not. x?=w91:bool)
                n54 = Build Array(w89, w90, w91) -> (w95:bool[])
                n55 = Boolean Array To Number(Boolean array=w95) -> (number=w197:u32)
                n56 = case shown="2" w197 {
                  frame 0, Default {
                    w523 = FALSE ("Confirma caminho 1")
                    n57 = property on="SKM-LAM-CTL" class="Bool (strict)"("Visible"=FALSE) -> ()  [unwired: 2 in, 2 out]
                    n58 = property on="SKM-FIC-COR-CTL" class="Bool (strict)"("Visible"=FALSE) -> ()  [unwired: 2 in, 2 out]
                    "Path" <- "Nenhum caminho escolhido" ("String 17")
                    "Confirma SKM-CV-COR" <- w523
                    "Confirma caminho 1" <- w523
                    "Confirma SKM-CV-LAM" <- w523
                  }
                  frame 1 {
                    w525 = FALSE ("AMS-EVC-001B")
                    n59 = local write "Confirma SKM-CV-LAM"(FALSE ("Confirma caminho 3")) -> ()
                    n60 = local write "Confirma SKM-CV-COR"(FALSE ("Confirma caminho 2")) -> ()
                    n61 = local write "Confirma caminho 1"(TRUE ("Confirma caminho 1")) -> ()
                    n62 = local write "AMS-EVC-001C"(w525) -> ()
                    n63 = local write "AMS-EVC-001B"(w525) -> ()
                    n64 = property on="SKM-LAM-CTL" class="Bool (strict)"("Visible"=FALSE) -> ()  [unwired: 2 in, 2 out]
                    n65 = property on="SKM-FIC-COR-CTL" class="Bool (strict)"("Visible"=TRUE) -> ()  [unwired: 2 in, 2 out]
                    n66 = local write "Path"("Laminador novo" ("Path")) -> ()
                  }
                  frame 2 {
                    w532 = FALSE ("AMS-EVC-001A")
                    n67 = local write "Confirma SKM-CV-LAM"(FALSE ("Confirma caminho 3")) -> ()
                    n68 = local write "Confirma SKM-CV-COR"(TRUE ("Confirma caminho 2")) -> ()
                    n69 = local write "Confirma caminho 1"(FALSE ("Confirma caminho 1")) -> ()
                    n70 = local write "AMS-EVC-001C"(w532) -> ()
                    n71 = local write "AMS-EVC-001A"(w532) -> ()
                    n72 = property on="SKM-LAM-CTL" class="Bool (strict)"("Visible"=TRUE) -> ()  [unwired: 2 in, 2 out]
                    n73 = property on="SKM-FIC-COR-CTL" class="Bool (strict)"("Visible"=FALSE) -> ()  [unwired: 2 in, 2 out]
                    n74 = local write "Path"("Coriolli" ("Path")) -> ()
                  }
                  frame 4 {
                    w539 = FALSE ("AMS-EVC-001A")
                    n75 = local write "AMS-EVC-001A"(w539) -> ()
                    n76 = local write "AMS-EVC-001B"(w539) -> ()
                    n77 = local write "Confirma SKM-CV-LAM"(TRUE ("Confirma caminho 3")) -> ()
                    n78 = local write "Confirma SKM-CV-COR"(FALSE ("Confirma caminho 2")) -> ()
                    n79 = local write "Confirma caminho 1"(FALSE ("Confirma caminho 1")) -> ()
                    n80 = property on="SKM-LAM-CTL" class="Bool (strict)"("Visible"=FALSE) -> ()  [unwired: 2 in, 2 out]
                    n81 = property on="SKM-FIC-COR-CTL" class="Bool (strict)"("Visible"=TRUE) -> ()  [unwired: 2 in, 2 out]
                    n82 = local write "Path"("Laminador" ("Path")) -> ()
                  }
                }
                n83 = call "Pump_Kerosene.vi"("Cluster_usuario_entrada_K"=w413, "todos_os_dados_ENTRADA"=w88, "todos_os_dados_SAIDA (controle)"=w414) -> ("Comparacao_server_skid_kerosene"=w402:T15, "TAG_para_PDF"=w433:string, "Cluster_usuario_saida_K"=w412:T16, "todos_os_dados_SAIDA (indicador)"=w437:T3, "Tipo de Dado"=w430:T2)  [unwired: 2 in]
                n84 = Unbundle By Name(w88) -> ("PAINEL_ADAM_ENTRADA.ANALOGICO.WPS-FCV-001-R"=→"WPS-FCV-001-R":dbl, "PAINEL_ADAM_ENTRADA.ANALOGICO.KPS-FCV-001-R"=→"KPS-FCV-001-R":dbl)
                n85 = call "Pump_Water.vi"("Cluster_usuario_entrada"=w199, "todos_os_dados_SAIDA"=w501, "todos_os_dados_ENTRADA"=w88) -> ("Comparacao_server_skid_agua"=w486:T17, "Cluster de usuario saida"=w487:T18, "todos_os_dados_SAIDA (indicador)"=w488:T3, "TAG_para_PDF"=w490:string, "Tipo de Dado"=w489:T2)  [unwired: 4 in]
                n86 = call "Skid_Medicao.vi"("Cluster_usuario_entrada"=w346, "todos_os_dados_SAIDA"=w348, "todos_os_dados_ENTRADA"=w88) -> ("Cluster_usuario_saida_medicao"=w388:T19, "Comparacao_server_skid_medicao"=w328:T20, "Tag_para_pdf_measure"=w432:string, "todos_os_dados_SAIDA (indicador)"=w435:T3, "Tipo de Dado"=w429:T2)  [unwired: 4 in]
                n87 = call "Skid_Injeção.vi"("Cluster de usuario_entrada"=w297, "padrao_todos_os_dados_ENTRADA"=w88, "todos_os_dados_SAIDA_C"=w321) -> ("Tag_para_pdf"=w431:string, "Tipo de Dado_I"=w428:T2, "Cluster de usuario_saida"=w320:T21, "todos_os_dados_SAIDA_I"=w434:T3, "Comparacao_server_skid_injecao"=w265:T22)  [unwired: 3 in]
                n88 = call "Skid_Separacao.vi"("todos_os_dados_ENTRADA"=w88, "path"=path "\\\\SERVERPC\\outros/Aplicacao_Super/main_super.vi" ("path 2"), "todos_os_dados_SAIDA (Controle)"=w257) -> ("todos_os_dados_SAIDA (Indicador)"=w436:T3, "Igual?Valvulas"=w216:T23, "Cluster de usuario (Indicador)"=w251:T24)  [unwired: 14 in]
                n89 = disable-structure shown="Disabled" {
                  frame Disabled {
                  }
                  frame Enabled {
                  }
                }
                n90 = Unbundle By Name(w328) -> ("igual?SKM-FC-AR"=→"igual?SKM-FC-AR":bool)
                n91 = Unbundle By Name(w487) -> ("Aux.WPS-FCV-001-AUX"=→"WPS-FCV-001-AUX":bool, "Tubos.T24"=→"T24":bool, "Tubos.T25"=→"T25":bool, "Tubos.T26"=→"T26":bool, "Tubos.T1"=→"T1":bool, "Tubos.T2"=→"T2":bool, "Tubos.T3"=→"T3":bool, "Tubos.T4"=→"T4":bool, "Tubos.T5"=→"T5":bool, "Tubos.T6"=→"T6":bool, "Tubos.T7"=→"T7":bool, "Tubos.T8"=→"T8":bool, "Tubos.T9"=→"T9":bool, "Tubos.T10"=→"T10":bool, "Tubos.T11"=→"T11":bool, "Tubos.T12"=→"T12":bool, "Tubos.T13"=→"T13":bool, "Tubos.T14"=→"T14":bool, "Tubos.T15"=→"T15":bool, "Tubos.T16"=→"T16":bool, "Tubos.T17"=→"T17":bool, "Tubos.T18"=→"T18":bool, "Tubos.T19"=→"T19":bool, "Tubos.T20"=→"T20":bool, "Tubos.T21"=→"T21":bool, "Tubos.T22"=→"T22":bool, "Tubos.T23"=→"T23":bool, "Inversor.Bomba"=→"Bomba W":bool, "Inversor.Inversor Ligado"=→"Inversor ligado":bool, "Inversor.Inversor Desligado"=→"Inversor desligado":bool, "Leitura_INV.SPW-RD-VEL"=w444:dbl, "Leitura_INV.SPW-RD-IA"=→"SPW-RD-IA":dbl, "Leitura_INV.SPW-RD-CRT"=→"SPW-RD-CRT":dbl, "Leitura_INV.SPW-RD-TU"=→"SPW-RD-TU":dbl, "Leitura_INV.SPW-PD-P"=→"SPW-PD-P":dbl, "Leitura_INV.SPW-RD-ST"=→"SPW-RD-ST":dbl)
                "SPW-RD-VEL" <- w444
                n92 = Unbundle By Name(w486) -> ("igual?SPW-CV-001"=→"igual?WPS-EVC-001":bool, "igual?SPW-CV-002"=→"igual?WPS-EVC-002":bool, "igual?SPW-CV-003"=→"igual?WPS-EVC-003":bool, "igual?SPW-CV-004"=→"igual?WPS-EVC-004":bool, "igual?SPW-CV-005"=→"igual?WPS-EVC-005":bool, "igual?SPW-CV-006"=→"igual?WPS-EVC-006":bool, "igual?SPW-CV-007"=→"igual?WPS-EVC-007":bool, "igual?SPW-CV-008"=→"igual?WPS-EVC-008":bool, "igual?SPW-WR-ON"=→"igual?SPW-WR-ON":bool, "igual?SPW-WR-OFF"=→"igual?SPW-WR-OFF":bool, "igual?PID-WF-ON"=→"igual?PID-WF-ON":bool, "igual?SPW-WR-VEL"=→"igual?SPW-WR-VEL":bool)
                n93 = Unbundle By Name(w388) -> ("Tubos.T49"=→"T49 M":bool, "Tubos.T1"=→"T1 M":bool, "Tubos.T2"=→"T2 M":bool, "Tubos.T3"=→"T3 M":bool, "Tubos.T4"=→"T4 M":bool, "Tubos.T5"=→"T5 M":bool, "Tubos.T6"=→"T6 M":bool, "Tubos.T7"=→"T7 M":bool, "Tubos.T8"=→"T8 M":bool, "Tubos.T9"=→"T9 M":bool, "Tubos.T10"=→"T10 M":bool, "Tubos.T11"=→"T11 M":bool, "Tubos.T12"=→"T12 M":bool, "Tubos.T13"=→"T13 M":bool, "Tubos.T14"=→"T14 M":bool, "Tubos.T15"=→"T15 M":bool, "Tubos.T16"=→"T16 M":bool, "Tubos.T17"=→"T17 M":bool, "Tubos.T18"=→"T18 M":bool, "Tubos.T19"=→"T19 M":bool, "Tubos.T20"=→"T20 M":bool, "Tubos.T21"=→"T21 M":bool, "Tubos.T22"=→"T22 M":bool, "Tubos.T23"=→"T23 M":bool, "Tubos.T24"=→"T24 M":bool, "Tubos.T25"=→"T25 M":bool, "Tubos.T26"=→"T26 M":bool, "Tubos.T27"=→"T27 M":bool, "Tubos.T28"=→"T28 M":bool, "Tubos.T29"=→"T29 M":bool, "Tubos.T30"=→"T30 M":bool, "Tubos.T31"=→"T31 M":bool, "Tubos.T32"=→"T32 M":bool, "Tubos.T33"=→"T33 M":bool, "Tubos.T34"=→"T34 M":bool, "Tubos.T35"=→"T35 M":bool, "Tubos.T36"=→"T36 M":bool, "Tubos.T37"=→"T37 M":bool, "Tubos.T38"=→"T38 M":bool, "Tubos.T39"=→"T39 M":bool, "Tubos.T40"=→"T40 M":bool, "Tubos.T41"=→"T41 M":bool, "Tubos.T42"=→"T42 M":bool, "Tubos.T43"=→"T43 M":bool, "Tubos.T44"=→"T44 M":bool, "Tubos.T45"=→"T45 M":bool, "Tubos.T46"=→"T46 M":bool, "Tubos.T47"=→"T47 M":bool, "Tubos.T48"=→"T48 M" →"aux1":bool, "Variaveis leitura rapida.AMS-PIT-003"=→"AMS-PIT-003":dbl[], "Variaveis leitura rapida.SKM-PA-LAM"=→"SKM-PA-LAM":dbl[], "Variaveis leitura rapida.SKM-TI-LAM"=→"SKM-TI-LAM":dbl[], "Variaveis leitura rapida.SKM-PD-LAM"=→"SKM-PD-LAM":dbl[], "Variaveis leitura rapida.WMS-FIT-TI-001A"=→"SKM-TI-COR-KF":dbl[], "Variaveis leitura rapida.WMS-FIT-DEN-001A"=→"SKM-DEN-COR-KF":dbl[], "Variaveis leitura rapida.WMS-FIT-FIC-001A"=→"SKM-FIC-COR-KF":dbl[], "Variaveis leitura rapida.KMS-FIT-TI-001"=→"SKM-TI-COR-AR":dbl[], "Variaveis leitura rapida.KMS-FIT-DEN-001"=→"SKM-DEN-COR-AR":dbl[], "Variaveis leitura rapida.KMS-FIT-FIC-001"=→"SKM-FIC-COR-AR":dbl[], "Variaveis leitura rapida.WMS-TIT-001"=→"WMS-TIT-001":dbl[], "Variaveis leitura rapida.KMS-TIT-002"=→"KMS-TIT-002":dbl[], "Variaveis leitura rapida.KMS-TIT-003"=→"KMS-TIT-003":dbl[], "Variaveis leitura rapida.WMS-FIT-001A"=→"WMS-FIT-001A":dbl[], "Variaveis leitura rapida.Vazao Massica Ar"=→"Vazao Massica Ar":dbl[], "Variaveis leitura rapida.SKM-PA-BAR"=→"SKM-PA-BAR":dbl[], "Aux.SKM-FC-WF-AUX"=→"SKM-FC-WF-AUX":bool, "Aux.SKM-FC-KF-AUX"=→"SKM-FC-KF-AUX":bool, "Aux.SKM-PC-TQ-AUX"=→"SKM-PC-TQ-AUX":bool, "Aux.SKM-FC-AR-AUX"=→"SKM-FC-AR-AUX":bool, "Aux.SKM-FIM-WF-CTL"=→"SKM-FIM-WF-CTL":bool, "Aux.SKM-FIC-COR-CTL"=→"SKM-FIC-COR-CTL":bool, "Aux.SKM-FIC-COR-KF-CTL"=→"SKM-FIC-COR-KF-CTL":bool, "Aux.SKM-LAM-CTL"=→"SKM-LAM-CTL":bool, "Aux.SKM-TI-KF-CTL"=→"SKM-TI-KF-CTL":bool, "Aux.SKM-TI-WF-CTL"=→"SKM-TI-WF-CTL":bool, "Variaveis leitura rapida.Temperatura"=→"Temperatura":dbl[], "Variaveis leitura rapida.Pressão Absoluta"=→"Pressao Absoluta":dbl[], "Variaveis leitura rapida.Pressão Diferencial"=→"Pressão Diferencial":dbl[])
                n94 = Unbundle By Name(w320) -> ("Tubos.T1"=→"T1 I":bool, "Tubos.T 2"=→"T2 I":bool, "Tubos.T 3"=→"T3 I":bool, "Tubos.T 4"=→"T4 I":bool, "Tubos.T 5"=→"T5 I":bool, "Tubos.T 6"=→"T6 I":bool, "Tubos.T 7"=→"T7 I":bool, "Tubos.T 8"=→"T8 I":bool, "Tubos.T 9"=→"T9 I":bool, "Tubos.T 10"=→"T10 I":bool, "Tubos.T 11"=→"T11 I":bool, "Tubos.T 12"=→"T12 I":bool, "Tubos.T 13"=→"T13 I":bool, "Tubos.T 14"=→"T14 I":bool, "Tubos.T 15"=→"T15 I":bool, "Tubos.T 16"=→"T16 I":bool, "Tubos.T 17"=→"T17 I":bool, "Tubos.T 18"=→"T18 I":bool, "Tubos.T 19"=→"T19 I":bool, "Tubos.T 20"=→"T20 I":bool, "Leitura.SKI-PD-ST"=→"SKI-PD-ST":dbl[])
                n95 = Unbundle By Name(w265) -> ("igual?SKI-CV-AR"=→"igual?SKI-CV-AR":bool, "igual?SKI-CV-KF-ST"=→"igual?SKI-CV-KF-ST":bool, "igual?SKI-CV-KF-BY1"=→"igual?SKI-CV-KF-BY1":bool, "igual?SKI-CV-WF-ST"=→"igual?SKI-CV-WF-ST":bool, "igual?SKI-CV-WF-BY1"=→"igual?SKI-CV-WF-BY1":bool, "igual?SKI-CV-ST"=→"igual?SKI-CV-ST":bool, "igual?SKI-CV-BY2"=→"igual?SKI-CV-BY2":bool)
                n96 = Unbundle By Name(w412) -> ("Tubos.T26"=→"T26 K":bool, "Tubos.T25"=→"T25 K":bool, "Tubos.T24"=→"T24 K":bool, "Tubos.T1"=→"T1 K":bool, "Tubos.T2"=→"T2 K":bool, "Tubos.T3"=→"T3 K":bool, "Tubos.T4"=→"T4 K":bool, "Tubos.T5"=→"T5 K":bool, "Tubos.T6"=→"T6 K":bool, "Tubos.T7"=→"T7 K":bool, "Tubos.T8"=→"T8 K":bool, "Tubos.T9"=→"T9 K":bool, "Tubos.T10"=→"T10 K":bool, "Tubos.T11"=→"T11 K":bool, "Tubos.T12"=→"T12 K":bool, "Tubos.T13"=→"T13 K":bool, "Tubos.T14"=→"T14 K":bool, "Tubos.T15"=→"T15 K":bool, "Tubos.T16"=→"T16 K":bool, "Tubos.T17"=→"T17 K":bool, "Tubos.T18"=→"T18 K":bool, "Tubos.T19"=→"T19 K":bool, "Tubos.T20"=→"T20 K":bool, "Tubos.T21"=→"T21 K":bool, "Tubos.T22"=→"T22 K":bool, "Tubos.T23"=→"T23 K":bool, "Leitura_INV.SPK-RD-ST"=→"SPK-RD-ST":dbl, "Leitura_INV.SPK-RD-VEL"=w266:dbl, "Leitura_INV.SPK-RD-IA"=→"SPK-RD-IA":dbl, "Leitura_INV.SPK-RD-CRT"=→"SPK-RD-CRT":dbl, "Leitura_INV.SPK-RD-TU"=→"SPK-RD-TU":dbl, "Leitura_INV.SPK-PD-P"=→"SPK-PD-P":dbl, "Inversor.Bomba"=→"Bomba K":bool, "Inversor.Inversor Ligado"=→"Inversor Ligado":bool, "Inversor.Inversor Desligado"=→"Inversor Desligado":bool, "Aux.SKM-FC-KF-AUX"=→"SKM-FC-KF-AUX 2":bool)
                "SPK-RD-VEL" <- w266
                n97 = Unbundle By Name(w402) -> ("igual?SPK-CV-001"=→"igual?SPK-CV-001":bool, "igual?SPK-CV-002"=→"igual?SPK-CV-002":bool, "igual?SPK-CV-003"=→"igual?SPK-CV-003":bool, "igual?SPK-CV-004"=→"igual?SPK-CV-004":bool, "igual?SPK-CV-005"=→"igual?SPK-CV-005":bool, "igual?SPK-CV-006"=→"igual?SPK-CV-006":bool, "igual?SPK-CV-007"=→"igual?SPK-CV-007":bool, "igual?SPK-CV-008"=→"igual?SPK-CV-008":bool, "igual?PID-KF-ON"=→"igual?PID-KF-ON":bool, "igual?SPK-WR-OFF"=→"igual?SPK-WR-OFF":bool, "igual?SPK-WR-ON"=→"igual?SPK-WR-ON":bool, "igual?SPK-WR-VEL"=→"igual?SPK-WR-VEL":bool)
                n98 = Unbundle By Name(w251) -> ("FSS-LSA-801"=→"FSS-LSA-801":bool, "FSS-LSA-621"=→"FSS-LSA-621":bool, "FSS-LSA-611"=→"FSS-LSA-611":bool, "FSS-LSL-621"=→"FSS-LSL-621":bool, "FSS-LSH-621"=→"FSS-LSH-621":bool, "FSS-LSL-611"=→"FSS-LSL-611":bool, "FSS-LSH-611"=→"FSS-LSH-611":bool, "TW2"=→"TW2":bool, "TK2"=→"TK2":bool, "TM5"=→"TM5":bool, "TM6"=→"TM6":bool, "TM7"=→"TM7":bool, "TM8"=→"TM8":bool, "TM9"=→"TM9":bool, "TM11"=→"TM11":bool, "FSS-LIT-801"=→"FSS-LIT-801":dbl, "FSS-LIT-802"=→"FSS-LIT-802":dbl, "TM10"=→"TM10":bool, "Valor minimo atingido K"=→"Minimo K":bool, "Valor maximo atingido K"=→"Maximo K":bool, "Valor maximo atingido W"=→"Maximo  W":bool, "Valor minimo atingido W"=→"Minimo  W":bool, "TK1"=→"TK1":bool, "TW3"=→"TW3":bool, "TW4"=→"TW4":bool, "TW5"=→"TW5":bool, "TW6"=→"TW6" →"aux2" →"aux3" →"aux4":bool, "TK3"=→"TK3":bool, "TK4"=→"TK4":bool, "TK5"=→"TK5":bool, "TK6"=→"TK6":bool, "TM4"=→"TM4":bool, "TW1"=→"TW1":bool, "FSS-EVC-621"=→"FSS-EVC-621":bool, "FSS-EVC-611"=→"FSS-EVC-611":bool, "TM1"=→"TM1":bool, "TM2"=→"TM2":bool, "TM3"=→"TM3":bool)
                n99 = Unbundle By Name(w216) -> ("Igual?SKS-CV-BY1"=→"igual?SKS-CV-BY1":bool, "Igual?SKS-CV-BY2"=→"igual?SKS-CV-BY2":bool, "Igual?SKS-CV-LT2"=→"igual?SKS-CV-LT2":bool, "Igual?SKS-CV-LT1"=→"igual?SKS-CV-LT1":bool)  [unwired: 2 out]
                n100 = Unbundle By Name(w88) -> ("UCM.004.EEL.0200_ENTRADA.DIGITAL.FSS-ZT-611"=w105:bool, "UCM.004.EEL.0200_ENTRADA.DIGITAL.FSS-ZT-621"=w104:bool)
                n101 = Unbundle By Name(w88) -> ("UCM.004.EEL.0300_ENTRADA.DIGITAL.AMS-ZT-001A"=w135:bool, "UCM.004.EEL.0300_ENTRADA.DIGITAL.AMS-ZT-001B"=w134:bool, "UCM.004.EEL.0300_ENTRADA.DIGITAL.AMS-ZT-001C"=w133:bool, "UCM.004.EEL.0300_ENTRADA.DIGITAL.AMS-ZT-003A"=w132:bool, "UCM.004.EEL.0300_ENTRADA.DIGITAL.WMS-ZT-001A"=w131:bool, "UCM.004.EEL.0300_ENTRADA.DIGITAL.KMS-ZT-001"=w130:bool, "UCM.004.EEL.0300_ENTRADA.DIGITAL.WMS-ZT-001B"=w113:bool)
                n102 = local read "AMS-EVC-003A"() -> (w119:bool)
                n103 = local read "AMS-EVC-001A"() -> (w128:bool)
                n104 = local read "AMS-EVC-001B"() -> (w126:bool)
                n105 = local read "AMS-EVC-001C"() -> (w124:bool)
                n106 = local read "WMS-EVC-001A"() -> (w115:bool)
                n107 = local read "KMS-EVC-001"() -> (w111:bool)
                n108 = local read "WMS-EVC-001B"() -> (w110:bool)
                n109 = Not(x=w105) -> (.not. x?=w103:bool)
                n110 = Not(x=w104) -> (.not. x?=w102:bool)
                n111 = local read "CP-Y-601H"() -> (w99:bool)
                n112 = local read "CP-Y-601D"() -> (w98:bool)
                n113 = Not(x=w135) -> (.not. x?=w129:bool)
                n114 = Not(x=w134) -> (.not. x?=w127:bool)
                n115 = Not(x=w133) -> (.not. x?=w125:bool)
                n116 = Not(x=w132) -> (.not. x?=w120:bool)
                n117 = Not(x=w131) -> (.not. x?=w114:bool)
                n118 = Not(x=w130) -> (.not. x?=w117:bool)
                n119 = Not(x=w113) -> (.not. x?=w112:bool)
                n120 = Divide(x=w266, y=3450.0) -> (x/y=w268:dbl)
                n121 = Divide(x=w444, y=3450.0) -> (x/y=w446:dbl)
                n122 = Multiply(x=w268, y=100.0) -> (x*y=→"SPK-RD-VEL[%]":dbl)
                n123 = Multiply(x=w446, y=100.0) -> (x*y=→"SPW-RD-VEL[%]":dbl)
                n124 = Equal?(x=w103, y=w99) -> (x = y?=→"igual?FSS-EVC-611":bool)
                n125 = Equal?(x=w102, y=w98) -> (x = y?=→"igual?FSS-EVC-621":bool)
                n126 = Equal?(x=w129, y=w128) -> (x = y?=→"igual?AMS-ECV-001A":bool)
                n127 = Equal?(x=w127, y=w126) -> (x = y?=→"igual?AMS-EVC-001B":bool)
                n128 = Equal?(x=w125, y=w124) -> (x = y?=→"igual?AMS-EVC-001C":bool)
                n129 = Equal?(x=w120, y=w119) -> (x = y?=→"igual?AMS-EVC-001E":bool)
                n130 = Equal?(x=w114, y=w115) -> (x = y?=→"igual?WMS-EVC-001A":bool)
                n131 = Equal?(x=w117, y=w111) -> (x = y?=→"igual?KMS-EVC-001":bool)
                n132 = Equal?(x=w112, y=w110) -> (x = y?=→"igual?WMS-EVC-001B":bool)
                n133 = call "Concatenador_tipo_dadoSuper.vi"("Tipo de Dado(SPW)"=w489, "Tipo de Dado(SPK)"=w430, "Tipo de Dado(SKM)"=w429, "Tipo de Dado(SKI)"=w428) -> ("Tipo de Dado(Final)"=w198:T2)  [unwired: 11 in]
                n134 = case shown="1" w198 {
                  frame 0, Default {
                    "SKM-FIC-COR-KF" <- "kg/s" ("String")
                    "SKM-TI-COR-KF" <- "ºC" ("String 2")
                    "SKM-DEN-COR-KF" <- "kg/m^3" ("String 3")
                    "SKM-TI-KF" <- "ºC" ("String 4")
                    "SKI-PD-ST" <- "" ("String 5")
                    "SKM-TI-WF" <- "ºC" ("String 6")
                    "SKM-FIM-WF" <- "m^3/s" ("String 7")
                    "SKM-PA-BAR" <- "kPa" ("String 8")
                    "SKM-TI-TQ" <- "ºC" ("String 9")
                    "SKM-PA-TQ" <- "kPa" ("String 10")
                    "Temp." <- "ºC" ("String 11")
                    "P.abs." <- "kPa" ("String 12")
                    "P.dif." <- "kPa" ("String 13")
                    "Vazao massica" <- "kg/s" ("String 15")
                  }
                  frame 1 {
                    n135 = local write "SKM-FIC-COR-KF"("Puro" ("String")) -> ()
                    n136 = local write "SKM-DEN-COR-KF"("Puro" ("String 3")) -> ()
                    n137 = local write "SKM-TI-COR-KF"("Puro" ("String 2")) -> ()
                    n138 = local write "SKM-PA-BAR"("Puro" ("String 8")) -> ()
                    n139 = local write "SKM-FIM-WF"("Puro" ("String 7")) -> ()
                    n140 = local write "SKM-TI-WF"("Puro" ("String 6")) -> ()
                    n141 = local write "SKM-TI-KF"("Puro" ("String 4")) -> ()
                    n142 = local write "SKI-PD-ST"("Puro" ("String 5")) -> ()
                    n143 = local write "SKM-TI-TQ"("Puro" ("String 9")) -> ()
                    n144 = local write "SKM-PA-TQ"("Puro" ("String 10")) -> ()
                    n145 = local write "Vazao massica"("Puro" ("String 15")) -> ()
                    n146 = local write "P.abs."("Puro" ("String 12")) -> ()
                    n147 = local write "P.dif."("Puro" ("String 13")) -> ()
                    n148 = local write "Temp."("Puro" ("String 11")) -> ()
                  }
                }
                n149 = call "Concatenador_tag_pdfSuper.vi"("TAG_PDF_SPW"=w490, "TAG_PDF_SPK"=w433, "TAG_PDF_SKM"=w432, "TAG_PDF_SKI"=w431) -> ("TAG_PDF_FINAL"=w503:string)  [unwired: 11 in]
                n150 = call "Concatenador_clusterSuper.vi"("todos_os_dados_SAIDA(SPW)"=w488, "todos_os_dados_SAIDA(SPK)"=w437, "todos_os_dados_SAIDA(SKM)"=w435, "todos_os_dados_SAIDA(SKI)"=w434, "todos_os_dados_SAIDA(SKS)"=w436) -> ("todos_os_dados_SAIDA(Final)"=w506:T3)  [unwired: 10 in]
                "Comunicacao Server Client" <- w507
                "Status_Comunicacao" <- w508
              }
              event "[ESC/STOP]": Value Change {
                w574 = FALSE ("Comunicacao Server Client")
                n151 = event-data() -> ("NewVal"=w577:bool)  [unwired: 1 in, 1 out]
                n152 = local write "Comunicacao Server Client"(w574) -> ()
                n153 = local write "RODANDO TESTE ??"(w574) -> ()
                n154 = invoke class="VI" method="Ctrl Val.Set"(reference=w580, error in=w579, "Control Name"="[ESC]", "Value"=w577) -> (reference out=w575:refnum<vi>, error out=w578:errorcluster)  [unwired: 1 in, 3 out]
                n155 = flat-sequence {
                  frame #0 {
                    w584 = FALSE ("SPW-CV-001")
                    w585 = i16 0 ("SKM-FC-KF")
                    w586 = FALSE ("SPW-CV-001")
                    w588 = FALSE ("SPW-CV-001")
                    w589 = FALSE ("SPW-CV-001")
                    w587 = FALSE ("SPW-CV-001")
                    w583 = FALSE ("SPW-CV-001")
                    # "SPW"
                    # "Voltando todas as valvulas para default apos encerrar os testes"
                    # "SKS"
                    # "SKI"
                    # "SKM-KEROSENE"
                    # "SKM-AGUA"
                    # "SKM-AR"
                    # "SPK"
                    n156 = local write "SPW-WR-VEL"(0 ("SPW-WR-VEL")) -> ()
                    n157 = local write "WPS-EVC-001"(w586) -> ()
                    n158 = local write "WPS-EVC-002"(w586) -> ()
                    n159 = local write "WPS-EVC-003"(w586) -> ()
                    n160 = local write "WPS-EVC-004"(w586) -> ()
                    n161 = local write "WPS-EVC-005"(w586) -> ()
                    n162 = local write "WPS-EVC-006"(w586) -> ()
                    n163 = local write "WPS-EVC-007"(w586) -> ()
                    n164 = local write "WPS-EVC-008"(w586) -> ()
                    n165 = local write "AMS-EVC-003A"(w584) -> ()
                    n166 = local write "KMS-EVC-001"(w584) -> ()
                    n167 = local write "WMS-EVC-001B"(w584) -> ()
                    n168 = local write "WMS-EVC-001A"(w584) -> ()
                    n169 = local write "AMS-EVC-001B"(w584) -> ()
                    n170 = local write "AMS-EVC-001C"(w584) -> ()
                    n171 = local write "AMS-EVC-001A"(w584) -> ()
                    n172 = local write "FIS-EVC-001"(w584) -> ()
                    n173 = local write "FIS-EVC-002"(w584) -> ()
                    n174 = local write "FIS-EVC-031"(w584) -> ()
                    n175 = local write "FIS-EVC-021"(w584) -> ()
                    n176 = local write "FIS-EVC-011"(w584) -> ()
                    n177 = local write "FIS-EVC-022"(w584) -> ()
                    n178 = local write "FIS-EVC-012"(w584) -> ()
                    n179 = local write "FSS-EVC-803"(w584) -> ()
                    n180 = local write "FSS-EVC-801"(w584) -> ()
                    n181 = local write "FSS-EVC-804"(w584) -> ()
                    n182 = local write "FSS-EVC-802"(w584) -> ()
                    n183 = local write "CP-Y-601D"(w584) -> ()
                    n184 = local write "CP-Y-601H"(w584) -> ()
                    n185 = local write "KPS-EVC-001"(w583) -> ()
                    n186 = local write "KPS-EVC-002"(w583) -> ()
                    n187 = local write "KPS-EVC-003"(w583) -> ()
                    n188 = local write "KPS-EVC-004"(w583) -> ()
                    n189 = local write "KPS-EVC-005"(w583) -> ()
                    n190 = local write "KPS-EVC-006"(w583) -> ()
                    n191 = local write "KPS-EVC-007"(w583) -> ()
                    n192 = local write "KPS-EVC-008"(w583) -> ()
                    n193 = local write "SPK-WR-VEL"(0 ("SPK-WR-VEL")) -> ()
                    n194 = local write "AMS-EVC-003A"(w587) -> ()
                    n195 = local write "AMS-EVC-001B"(w587) -> ()
                    n196 = local write "AMS-EVC-001C"(w587) -> ()
                    n197 = local write "AMS-FY-004A"(i16 0 ("SKM-FC-AR")) -> ()
                    n198 = local write "AMS-PY-005A"(i16 0 ("SKM-PC-TQ")) -> ()
                    n199 = local write "WPS-FCV-001-W"(w585) -> ()
                    n200 = local write "KPS-FCV-001-W"(w585) -> ()
                    n201 = local write "KMS-FCV-001"(i16 0 ("SKM-FC-KF")) -> ()
                    n202 = local write "WMS-FCV-001"(i16 0 ("SKM-FC-WF")) -> ()
                    n203 = local write "FIS-EVC-001"(w589) -> ()
                    n204 = local write "FIS-EVC-031"(w589) -> ()
                    n205 = local write "FIS-EVC-002"(w589) -> ()
                    n206 = local write "FIS-EVC-011"(w589) -> ()
                    n207 = local write "FIS-EVC-021"(w589) -> ()
                    n208 = local write "FIS-EVC-012"(w589) -> ()
                    n209 = local write "FIS-EVC-022"(w589) -> ()
                    n210 = local write "FSS-EVC-801"(w588) -> ()
                    n211 = local write "FSS-EVC-803"(w588) -> ()
                    n212 = local write "FSS-EVC-804"(w588) -> ()
                    n213 = local write "FSS-EVC-802"(w588) -> ()
                    n214 = local write "CP-Y-601H"(w588) -> ()
                    n215 = local write "CP-Y-601D"(w588) -> ()
                  }
                  frame #1 {
                    n216 = Wait (ms)(milliseconds to wait=u32 100) -> ()  [unwired: 1 out]
                  }
                }
              }
            }
            n217 = call "Bloco_escritaSuper.vi"("reference"=w74, "error in (no error)"=w71, "Tag_para_PDF"=w76, "Tipo de Dado"=w69, "Abrir Editor Prioridade"=w75, "todos_os_dados_SAIDA"=w70) -> ("reference out"=w73:refnum<vi>, "error out"=w72:errorcluster)  [unwired: 12 in]
          }
        }
      }
    }
  }
  n218 = call "Abort_super.vi"("reference"=w2, "error in (no error)"=w10) -> ()  [unwired: 9 in]
